vi "Experiment 19.vi"() -> ()   [LabVIEW 2026]
doc: "Experiment 19\nThis experiment is like Experiment 12 but contains 14 parallel loops (instead of 10 as in Exp 12)."
uses:
  <vilib>/AdvancedString/1D String Array to Delimited String (string).vi
  <vilib>/Analysis/baseanly.llb/Mean (DBL).vi
  <vilib>/Analysis/NI_AALBase.lvlib
panel:
  out "No. Of Iterations Executed - Loop 14":i32
  out "Output - Loop 14":dbl[](array[numeric]) format="%.3f"
  out "No. Of Iterations Executed - Loop 13":i32
  out "Output - Loop 13":dbl[](array[numeric]) format="%.3f"
  out "No. Of Iterations Executed - Loop 12":i32
  out "Output - Loop 12":dbl[](array[numeric]) format="%.3f"
  out "No. Of Iterations Executed - Loop 11":i32
  out "Output - Loop 11":dbl[](array[numeric]) format="%.3f"
  out "No. Of Iterations As Block Of Text (easy to copy into Excel)":string
  out "No. Of Iterations Executed - Loop 10":i32
  out "Output - Loop 10":dbl[](array[numeric]) format="%.3f"
  out "No. Of Iterations Executed - Loop 9":i32
  out "Output - Loop 9":dbl[](array[numeric]) format="%.3f"
  out "No. Of Iterations Executed - Loop 8":i32
  out "Output - Loop 8":dbl[](array[numeric]) format="%.3f"
  out "No. Of Iterations Executed - Loop 7":i32
  out "Output - Loop 7":dbl[](array[numeric]) format="%.3f"
  out "No. Of Iterations Executed - Loop 6":i32
  out "Output - Loop 6":dbl[](array[numeric]) format="%.3f"
  out "No. Of Iterations Executed - Loop 5":i32
  out "Output - Loop 5":dbl[](array[numeric]) format="%.3f"
  out "No. Of Iterations Executed - Loop 4":i32
  out "Output - Loop 4":dbl[](array[numeric]) format="%.3f"
  out "No. Of Iterations Executed - Loop 3":i32
  out "Output - Loop 3":dbl[](array[numeric]) format="%.3f"
  out "Avg. No. Of Iterations Executed - All Loops":dbl format="%.1f"
  out "No. Of Iterations Executed - Loop 2":i32
  out "Output - Loop 2":dbl[](array[numeric]) format="%.3f"
  out "No. Of Iterations Executed - Loop 1":i32
  out "Output - Loop 1":dbl[](array[numeric]) format="%.3f"
  out "Stop VI?":bool
  # "Experiment 19"
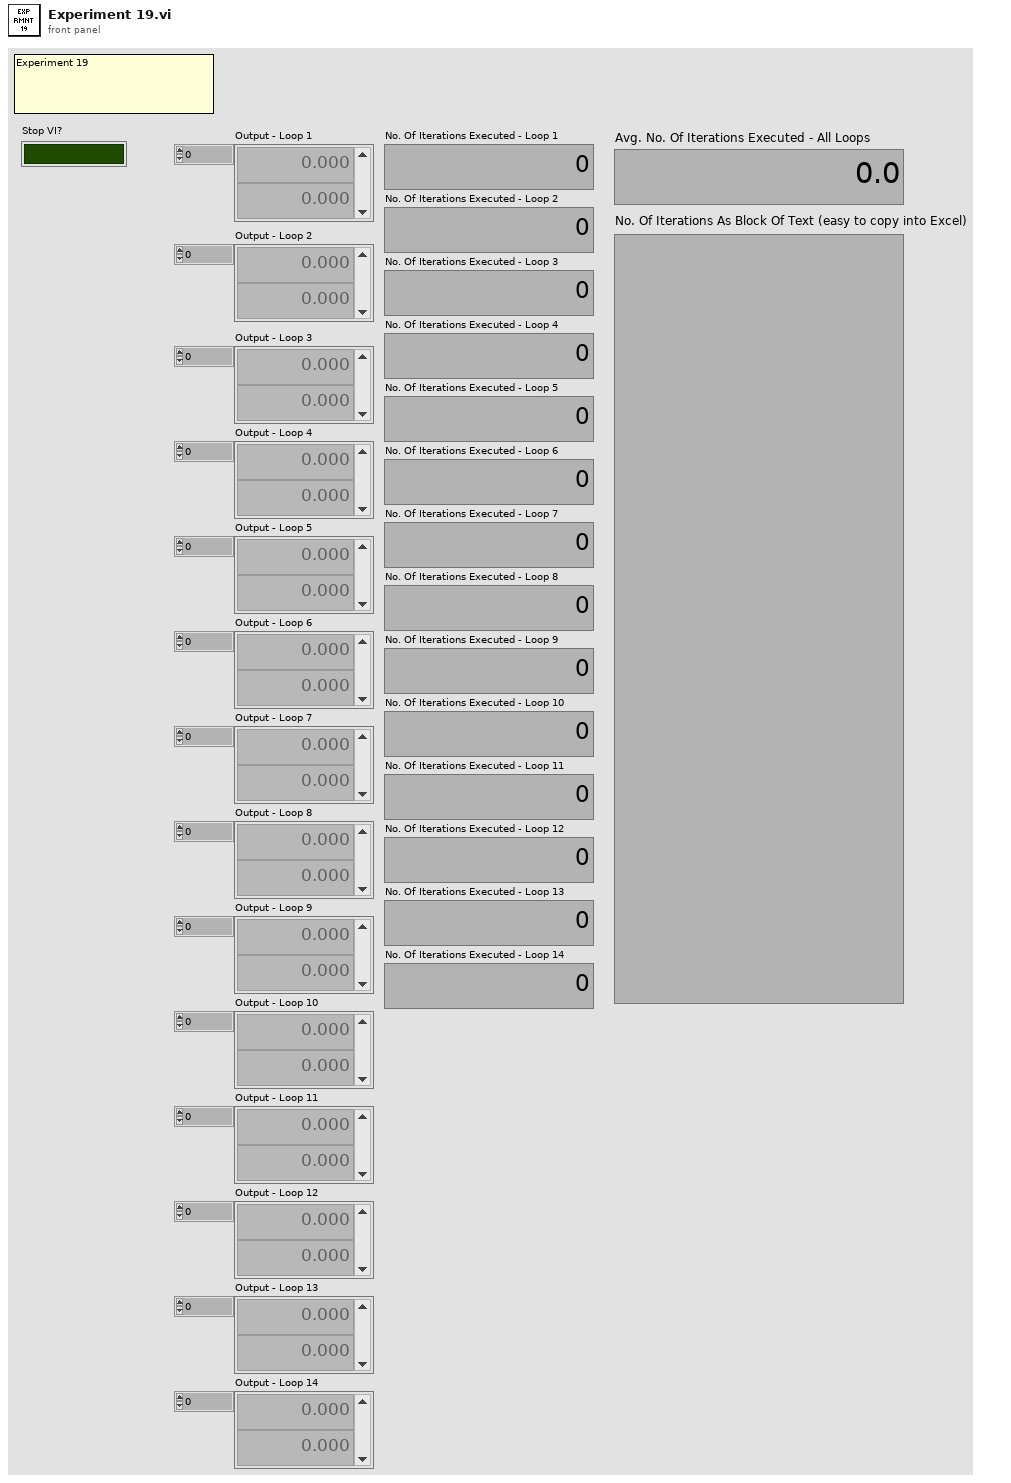
[diagram p1: front panel]
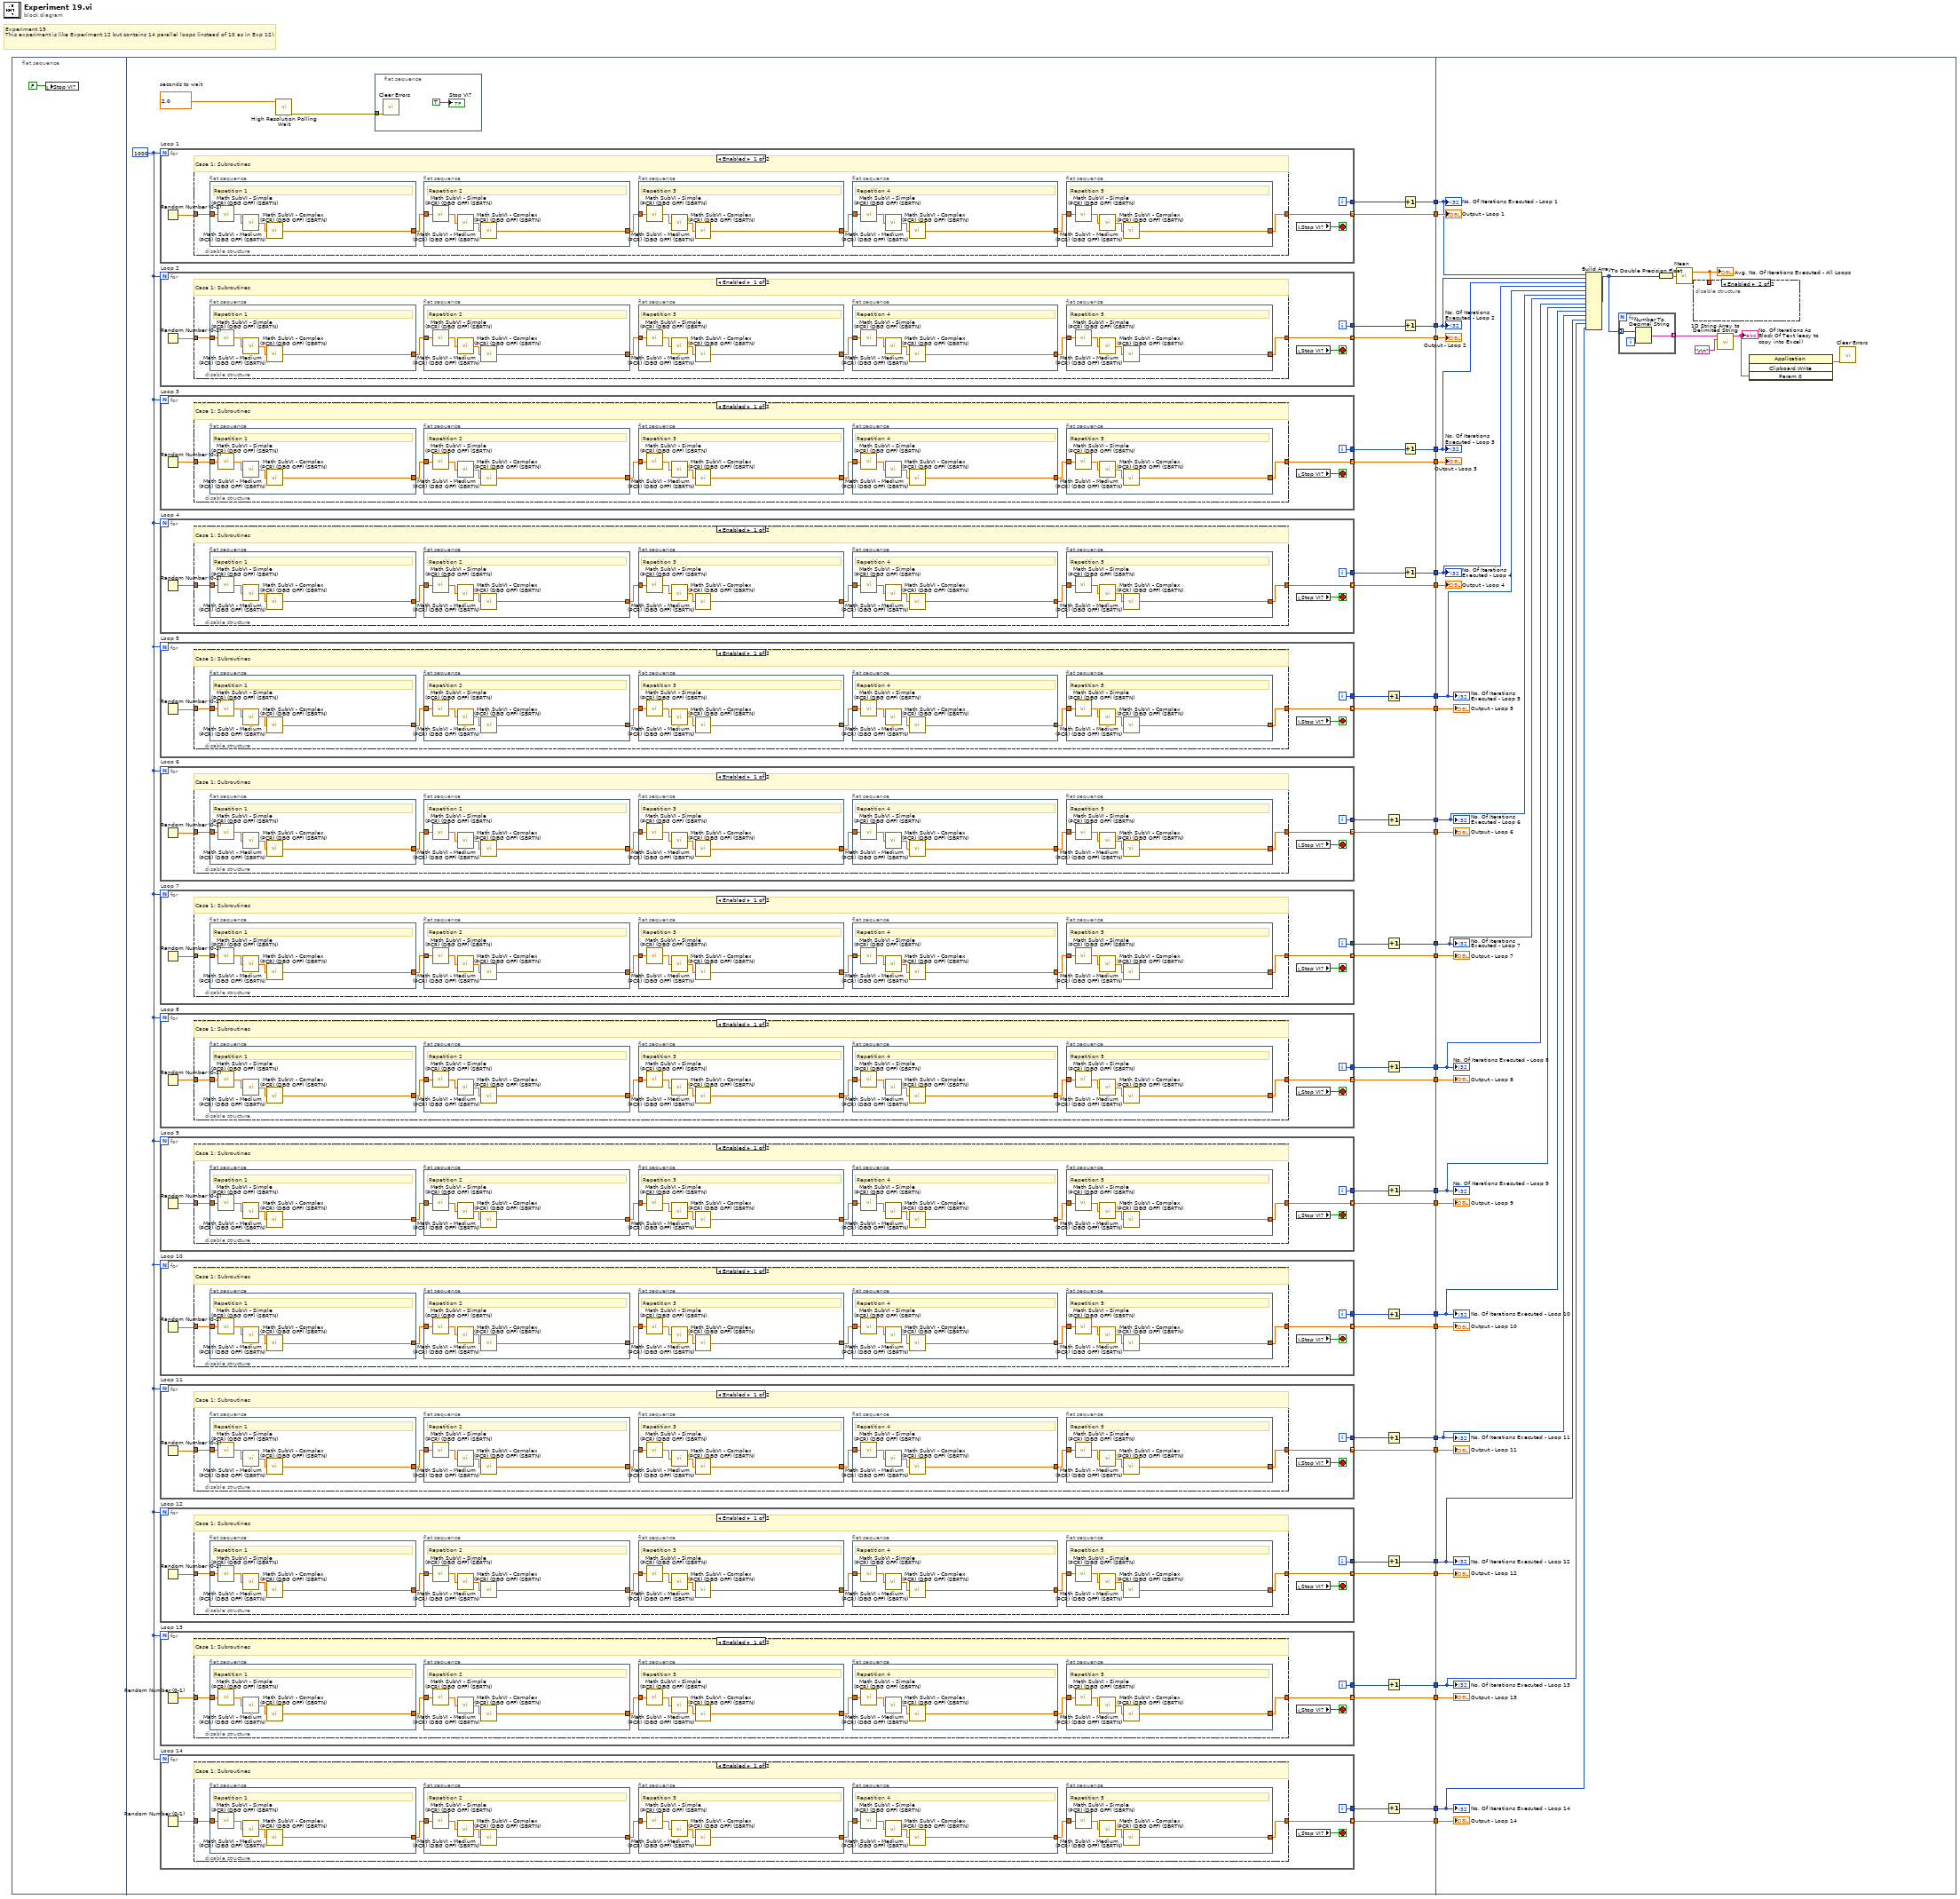
[diagram p0: block diagram]
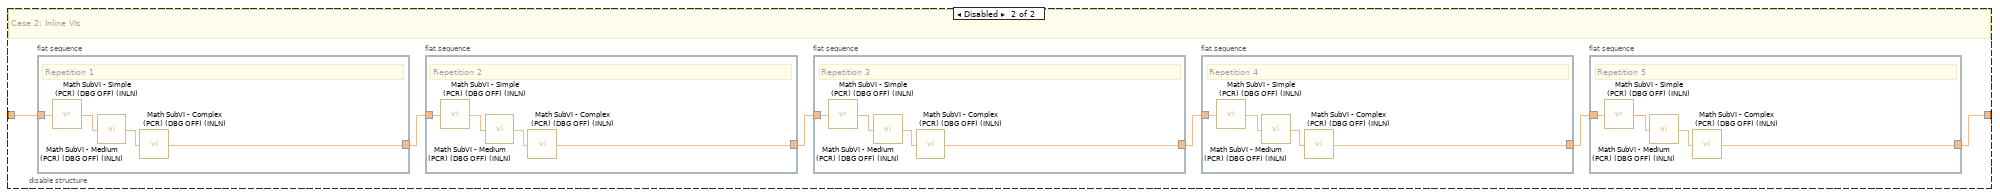
[diagram p2: hidden frame]
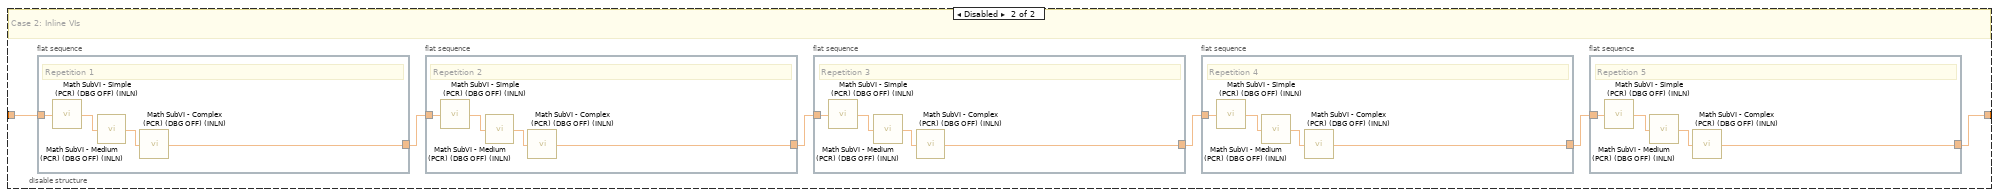
[diagram p3: hidden frame]
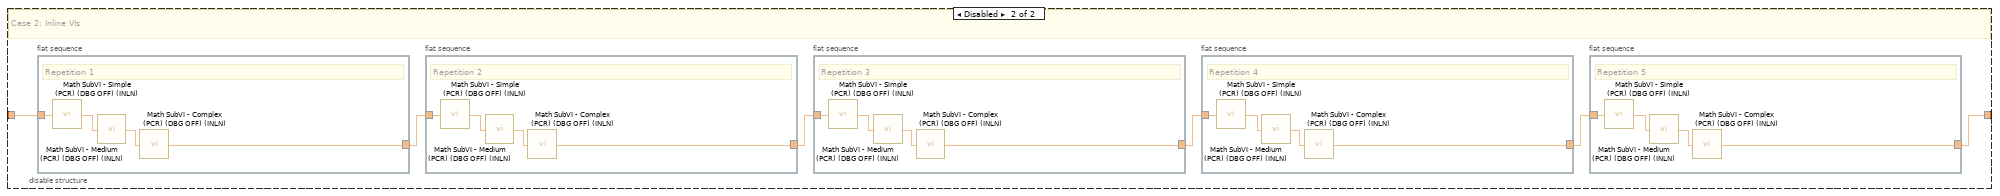
[diagram p4: hidden frame]
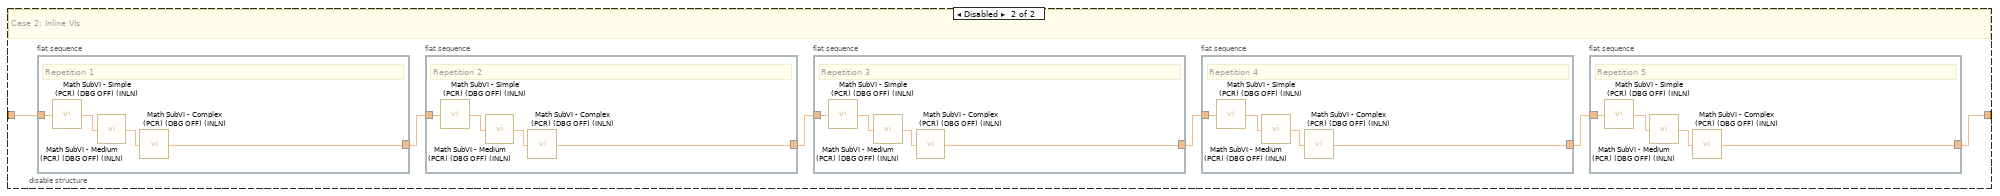
[diagram p5: hidden frame]
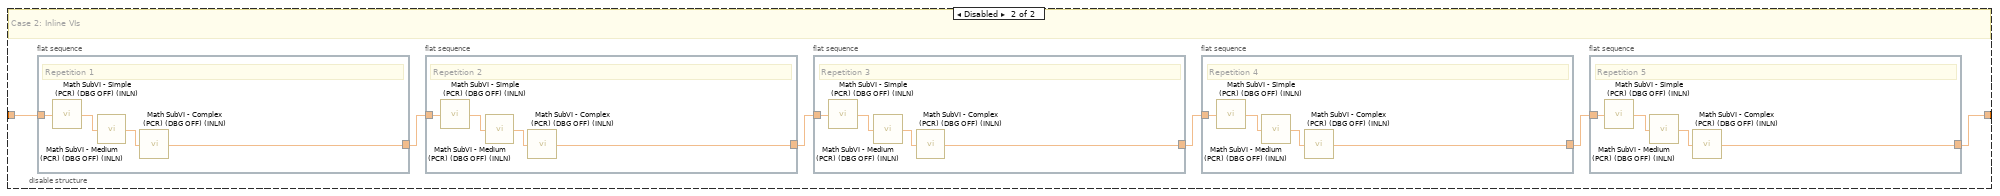
[diagram p6: hidden frame]
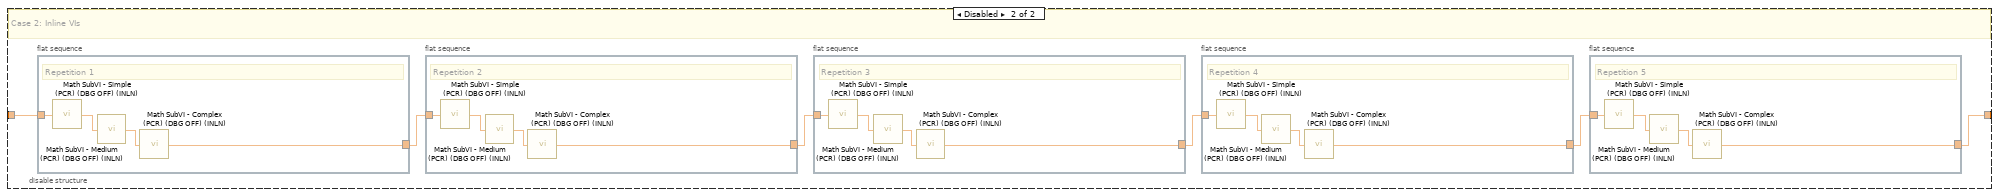
[diagram p7: hidden frame]
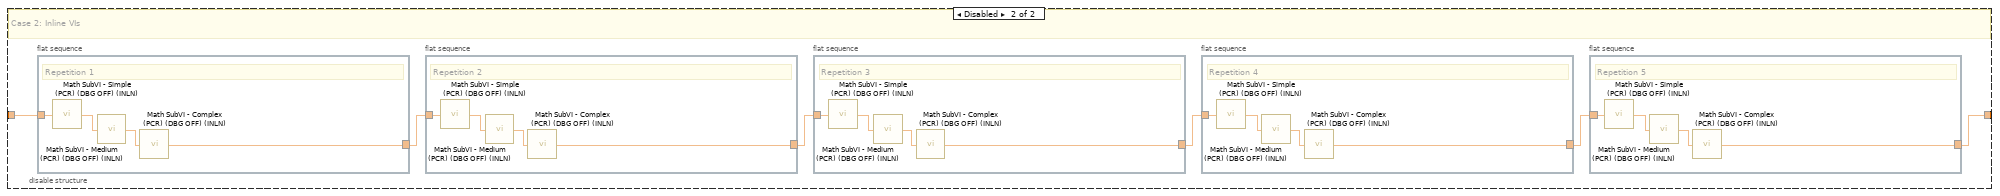
[diagram p8: hidden frame]
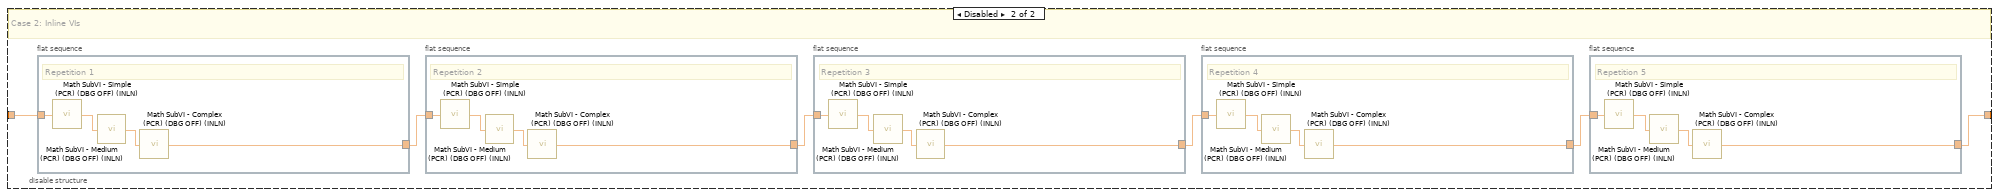
[diagram p9: hidden frame]
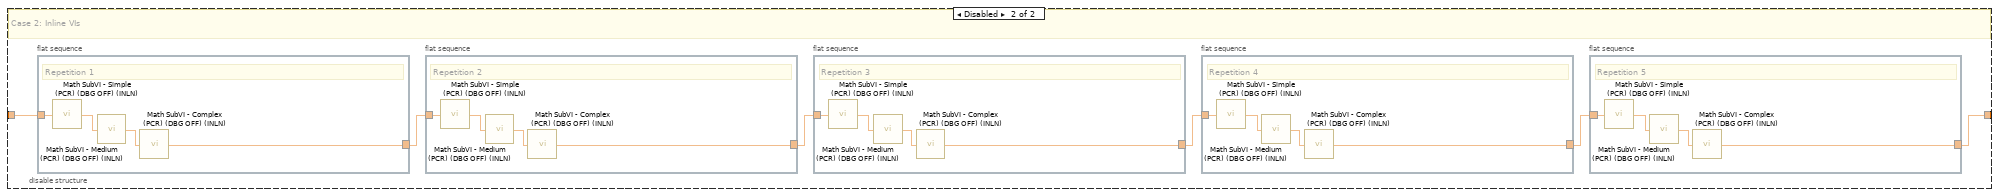
[diagram p10: hidden frame]
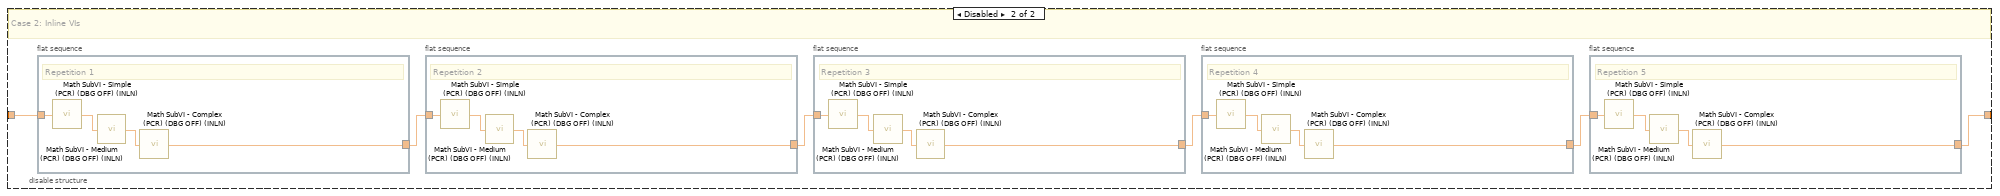
[diagram p11: hidden frame]
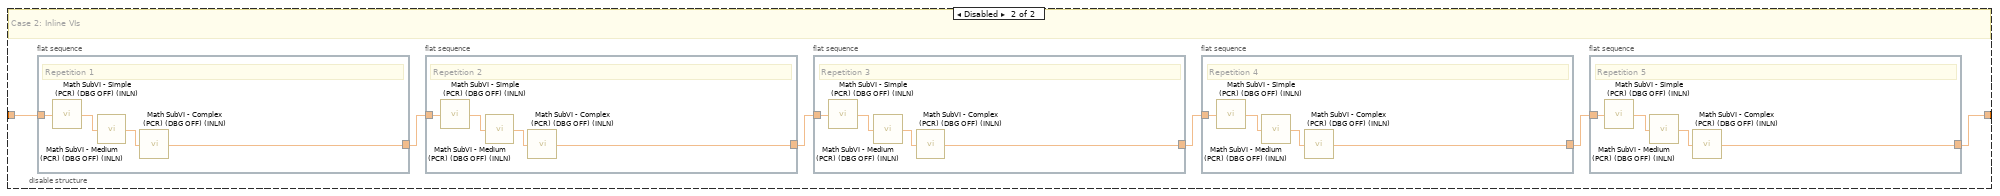
[diagram p12: hidden frame]
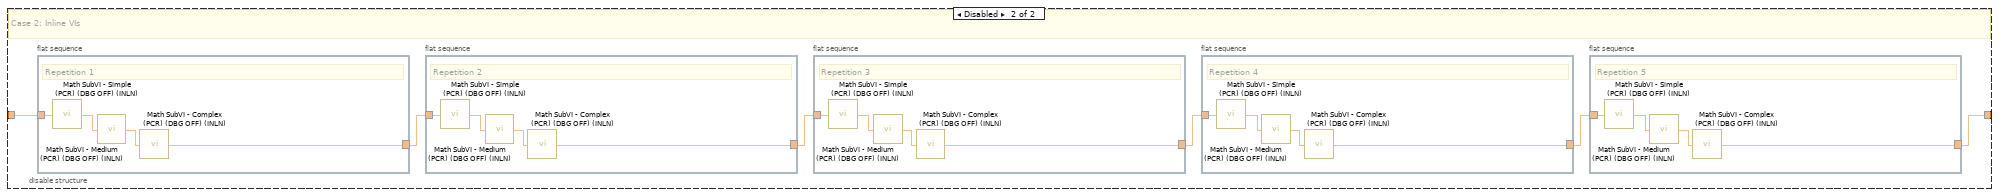
[diagram p13: hidden frame]
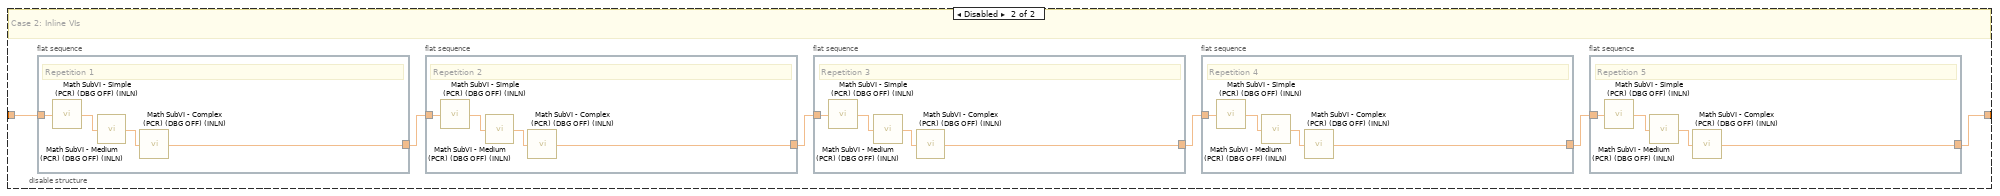
[diagram p14: hidden frame]
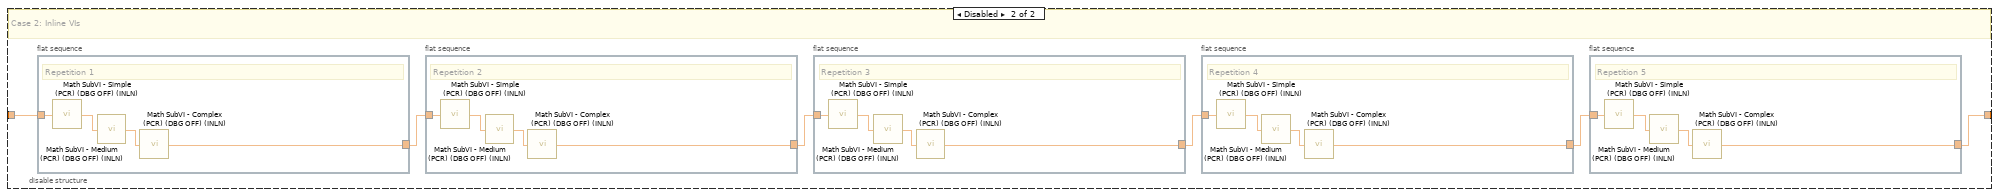
[diagram p15: hidden frame]
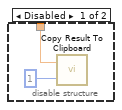
[diagram p16: hidden frame]
diagram:
  # "Experiment 19\nThis experiment is like Experiment 12 but contains 14 parallel loops (instead of 10 as in Exp 12)."
  n1 = flat-sequence {
    tunnel: [w72] -> w28
    tunnel: [w70] -> w27
    tunnel: [w69] -> w26
    tunnel: [w60] -> w25
    tunnel: [w68] -> w24
    tunnel: [w58] -> w23
    tunnel: [w56] -> w22
    tunnel: [w67] -> w21
    tunnel: [w54] -> w20
    tunnel: [w66] -> w19
    tunnel: [w52] -> w18
    tunnel: [w61] -> w17
    tunnel: [w50] -> w16
    tunnel: [w62] -> w15
    tunnel: [w47] -> w14
    tunnel: [w63] -> w13
    tunnel: [w45] -> w12
    tunnel: [w64] -> w11
    tunnel: [w43] -> w10
    tunnel: [w65] -> w9
    tunnel: [w41] -> w8
    tunnel: [w39] -> w7
    tunnel: [w38] -> w6
    tunnel: [w32] -> w5
    tunnel: [w36] -> w4
    tunnel: [w31] -> w3
    tunnel: [w34] -> w2
    tunnel: [w30] -> w1
    tunnel: w28 -> [w895]
    tunnel: w27 -> [w893]
    tunnel: w26 -> [w892]
    tunnel: w25 -> [w894]
    tunnel: w24 -> [w888]
    tunnel: w23 -> [w890]
    tunnel: w22 -> [w889]
    tunnel: w21 -> [w887]
    tunnel: w20 -> [w885]
    tunnel: w19 -> [w879]
    tunnel: w18 -> [w884]
    tunnel: w17 -> [w878]
    tunnel: w16 -> [w883]
    tunnel: w15 -> [w877]
    tunnel: w14 -> [w882]
    tunnel: w13 -> [w876]
    tunnel: w12 -> [w881]
    tunnel: w11 -> [w875]
    tunnel: w10 -> [w880]
    tunnel: w9 -> [w874]
    tunnel: w8 -> [w868]
    tunnel: w7 -> [w864]
    tunnel: w6 -> [w867]
    tunnel: w5 -> [w863]
    tunnel: w4 -> [w866]
    tunnel: w3 -> [w862]
    tunnel: w2 -> [w865]
    tunnel: w1 -> [w861]
    frame #0 {
      n2 = local write "Stop VI?"(FALSE) -> ()
    }
    frame #1 {
      w42 = 10000000
      w74 = 2.0  # seconds to wait
      n3 = for "Loop 1" {
        N: w42 -> [_]
        tunnel: [w806] -> w72 mode=indexing
        tunnel: [w807] -> w71
        i -> [w807]
        stop <- w808 stop-if-true
        n4 = Random Number (0-1)() -> (number: 0 to 1=w805:dbl)
        n5 = disable-structure shown="Enabled" {
          disable-tunnel: w805 -> [w814 w840]
          disable-tunnel: [w813 w835] -> w806
          frame Enabled {
            # "Case 1: Subroutines"
            n6 = flat-sequence {
              tunnel: w814 -> [w834]
              tunnel: [w831] -> w809
              frame #0 {
                # "Repetition 1"
                n7 = call "Math SubVI - Simple (PCR) (DBG OFF) (SBRTN).vi"("Input"=w834) -> ("Output"=w832:dbl)
                n8 = call "Math SubVI - Medium (PCR) (DBG OFF) (SBRTN).vi"("Input"=w832) -> ("Output"=w833:dbl)
                n9 = call "Math SubVI - Complex (PCR) (DBG OFF) (SBRTN).vi"("Input"=w833) -> ("Output"=w831:dbl)
              }
            }
            n10 = flat-sequence {
              tunnel: w809 -> [w830]
              tunnel: [w827] -> w812
              frame #0 {
                # "Repetition 2"
                n11 = call "Math SubVI - Simple (PCR) (DBG OFF) (SBRTN).vi"("Input"=w830) -> ("Output"=w828:dbl)
                n12 = call "Math SubVI - Medium (PCR) (DBG OFF) (SBRTN).vi"("Input"=w828) -> ("Output"=w829:dbl)
                n13 = call "Math SubVI - Complex (PCR) (DBG OFF) (SBRTN).vi"("Input"=w829) -> ("Output"=w827:dbl)
              }
            }
            n14 = flat-sequence {
              tunnel: w812 -> [w826]
              tunnel: [w823] -> w811
              frame #0 {
                # "Repetition 3"
                n15 = call "Math SubVI - Simple (PCR) (DBG OFF) (SBRTN).vi"("Input"=w826) -> ("Output"=w824:dbl)
                n16 = call "Math SubVI - Medium (PCR) (DBG OFF) (SBRTN).vi"("Input"=w824) -> ("Output"=w825:dbl)
                n17 = call "Math SubVI - Complex (PCR) (DBG OFF) (SBRTN).vi"("Input"=w825) -> ("Output"=w823:dbl)
              }
            }
            n18 = flat-sequence {
              tunnel: w811 -> [w822]
              tunnel: [w819] -> w810
              frame #0 {
                # "Repetition 4"
                n19 = call "Math SubVI - Simple (PCR) (DBG OFF) (SBRTN).vi"("Input"=w822) -> ("Output"=w820:dbl)
                n20 = call "Math SubVI - Medium (PCR) (DBG OFF) (SBRTN).vi"("Input"=w820) -> ("Output"=w821:dbl)
                n21 = call "Math SubVI - Complex (PCR) (DBG OFF) (SBRTN).vi"("Input"=w821) -> ("Output"=w819:dbl)
              }
            }
            n22 = flat-sequence {
              tunnel: w810 -> [w818]
              tunnel: [w815] -> w813
              frame #0 {
                # "Repetition 5"
                n23 = call "Math SubVI - Simple (PCR) (DBG OFF) (SBRTN).vi"("Input"=w818) -> ("Output"=w816:dbl)
                n24 = call "Math SubVI - Medium (PCR) (DBG OFF) (SBRTN).vi"("Input"=w816) -> ("Output"=w817:dbl)
                n25 = call "Math SubVI - Complex (PCR) (DBG OFF) (SBRTN).vi"("Input"=w817) -> ("Output"=w815:dbl)
              }
            }
          }
          frame Disabled {
            # "Case 2: Inline VIs"
            n26 = flat-sequence {
              tunnel: w840 -> [w860]
              tunnel: [w857] -> w839
              frame #0 {
                # "Repetition 1"
                n27 = call "Math SubVI - Simple (PCR) (DBG OFF) (INLN).vi"("Input"=w860) -> ("Output"=w858:dbl)
                n28 = call "Math SubVI - Medium (PCR) (DBG OFF) (INLN).vi"("Input"=w858) -> ("Output"=w859:dbl)
                n29 = call "Math SubVI - Complex (PCR) (DBG OFF) (INLN).vi"("Input"=w859) -> ("Output"=w857:dbl)
              }
            }
            n30 = flat-sequence {
              tunnel: w839 -> [w856]
              tunnel: [w853] -> w838
              frame #0 {
                # "Repetition 2"
                n31 = call "Math SubVI - Simple (PCR) (DBG OFF) (INLN).vi"("Input"=w856) -> ("Output"=w854:dbl)
                n32 = call "Math SubVI - Medium (PCR) (DBG OFF) (INLN).vi"("Input"=w854) -> ("Output"=w855:dbl)
                n33 = call "Math SubVI - Complex (PCR) (DBG OFF) (INLN).vi"("Input"=w855) -> ("Output"=w853:dbl)
              }
            }
            n34 = flat-sequence {
              tunnel: w838 -> [w852]
              tunnel: [w849] -> w837
              frame #0 {
                # "Repetition 3"
                n35 = call "Math SubVI - Simple (PCR) (DBG OFF) (INLN).vi"("Input"=w852) -> ("Output"=w850:dbl)
                n36 = call "Math SubVI - Medium (PCR) (DBG OFF) (INLN).vi"("Input"=w850) -> ("Output"=w851:dbl)
                n37 = call "Math SubVI - Complex (PCR) (DBG OFF) (INLN).vi"("Input"=w851) -> ("Output"=w849:dbl)
              }
            }
            n38 = flat-sequence {
              tunnel: w837 -> [w848]
              tunnel: [w845] -> w836
              frame #0 {
                # "Repetition 4"
                n39 = call "Math SubVI - Simple (PCR) (DBG OFF) (INLN).vi"("Input"=w848) -> ("Output"=w846:dbl)
                n40 = call "Math SubVI - Medium (PCR) (DBG OFF) (INLN).vi"("Input"=w846) -> ("Output"=w847:dbl)
                n41 = call "Math SubVI - Complex (PCR) (DBG OFF) (INLN).vi"("Input"=w847) -> ("Output"=w845:dbl)
              }
            }
            n42 = flat-sequence {
              tunnel: w836 -> [w844]
              tunnel: [w841] -> w835
              frame #0 {
                # "Repetition 5"
                n43 = call "Math SubVI - Simple (PCR) (DBG OFF) (INLN).vi"("Input"=w844) -> ("Output"=w842:dbl)
                n44 = call "Math SubVI - Medium (PCR) (DBG OFF) (INLN).vi"("Input"=w842) -> ("Output"=w843:dbl)
                n45 = call "Math SubVI - Complex (PCR) (DBG OFF) (INLN).vi"("Input"=w843) -> ("Output"=w841:dbl)
              }
            }
          }
        }
        n46 = local read "Stop VI?"() -> (w808:bool)
      }
      n47 = for "Loop 2" {
        N: w42 -> [_]
        tunnel: [w750] -> w60 mode=indexing
        tunnel: [w751] -> w59
        i -> [w751]
        stop <- w752 stop-if-true
        n48 = Random Number (0-1)() -> (number: 0 to 1=w749:dbl)
        n49 = disable-structure shown="Enabled" {
          disable-tunnel: w749 -> [w758 w784]
          disable-tunnel: [w757 w779] -> w750
          frame Enabled {
            # "Case 1: Subroutines"
            n50 = flat-sequence {
              tunnel: w758 -> [w778]
              tunnel: [w775] -> w753
              frame #0 {
                # "Repetition 1"
                n51 = call "Math SubVI - Simple (PCR) (DBG OFF) (SBRTN).vi"("Input"=w778) -> ("Output"=w776:dbl)
                n52 = call "Math SubVI - Medium (PCR) (DBG OFF) (SBRTN).vi"("Input"=w776) -> ("Output"=w777:dbl)
                n53 = call "Math SubVI - Complex (PCR) (DBG OFF) (SBRTN).vi"("Input"=w777) -> ("Output"=w775:dbl)
              }
            }
            n54 = flat-sequence {
              tunnel: w753 -> [w774]
              tunnel: [w771] -> w756
              frame #0 {
                # "Repetition 2"
                n55 = call "Math SubVI - Simple (PCR) (DBG OFF) (SBRTN).vi"("Input"=w774) -> ("Output"=w772:dbl)
                n56 = call "Math SubVI - Medium (PCR) (DBG OFF) (SBRTN).vi"("Input"=w772) -> ("Output"=w773:dbl)
                n57 = call "Math SubVI - Complex (PCR) (DBG OFF) (SBRTN).vi"("Input"=w773) -> ("Output"=w771:dbl)
              }
            }
            n58 = flat-sequence {
              tunnel: w756 -> [w770]
              tunnel: [w767] -> w755
              frame #0 {
                # "Repetition 3"
                n59 = call "Math SubVI - Simple (PCR) (DBG OFF) (SBRTN).vi"("Input"=w770) -> ("Output"=w768:dbl)
                n60 = call "Math SubVI - Medium (PCR) (DBG OFF) (SBRTN).vi"("Input"=w768) -> ("Output"=w769:dbl)
                n61 = call "Math SubVI - Complex (PCR) (DBG OFF) (SBRTN).vi"("Input"=w769) -> ("Output"=w767:dbl)
              }
            }
            n62 = flat-sequence {
              tunnel: w755 -> [w766]
              tunnel: [w763] -> w754
              frame #0 {
                # "Repetition 4"
                n63 = call "Math SubVI - Simple (PCR) (DBG OFF) (SBRTN).vi"("Input"=w766) -> ("Output"=w764:dbl)
                n64 = call "Math SubVI - Medium (PCR) (DBG OFF) (SBRTN).vi"("Input"=w764) -> ("Output"=w765:dbl)
                n65 = call "Math SubVI - Complex (PCR) (DBG OFF) (SBRTN).vi"("Input"=w765) -> ("Output"=w763:dbl)
              }
            }
            n66 = flat-sequence {
              tunnel: w754 -> [w762]
              tunnel: [w759] -> w757
              frame #0 {
                # "Repetition 5"
                n67 = call "Math SubVI - Simple (PCR) (DBG OFF) (SBRTN).vi"("Input"=w762) -> ("Output"=w760:dbl)
                n68 = call "Math SubVI - Medium (PCR) (DBG OFF) (SBRTN).vi"("Input"=w760) -> ("Output"=w761:dbl)
                n69 = call "Math SubVI - Complex (PCR) (DBG OFF) (SBRTN).vi"("Input"=w761) -> ("Output"=w759:dbl)
              }
            }
          }
          frame Disabled {
            # "Case 2: Inline VIs"
            n70 = flat-sequence {
              tunnel: w784 -> [w804]
              tunnel: [w801] -> w783
              frame #0 {
                # "Repetition 1"
                n71 = call "Math SubVI - Simple (PCR) (DBG OFF) (INLN).vi"("Input"=w804) -> ("Output"=w802:dbl)
                n72 = call "Math SubVI - Medium (PCR) (DBG OFF) (INLN).vi"("Input"=w802) -> ("Output"=w803:dbl)
                n73 = call "Math SubVI - Complex (PCR) (DBG OFF) (INLN).vi"("Input"=w803) -> ("Output"=w801:dbl)
              }
            }
            n74 = flat-sequence {
              tunnel: w783 -> [w800]
              tunnel: [w797] -> w782
              frame #0 {
                # "Repetition 2"
                n75 = call "Math SubVI - Simple (PCR) (DBG OFF) (INLN).vi"("Input"=w800) -> ("Output"=w798:dbl)
                n76 = call "Math SubVI - Medium (PCR) (DBG OFF) (INLN).vi"("Input"=w798) -> ("Output"=w799:dbl)
                n77 = call "Math SubVI - Complex (PCR) (DBG OFF) (INLN).vi"("Input"=w799) -> ("Output"=w797:dbl)
              }
            }
            n78 = flat-sequence {
              tunnel: w782 -> [w796]
              tunnel: [w793] -> w781
              frame #0 {
                # "Repetition 3"
                n79 = call "Math SubVI - Simple (PCR) (DBG OFF) (INLN).vi"("Input"=w796) -> ("Output"=w794:dbl)
                n80 = call "Math SubVI - Medium (PCR) (DBG OFF) (INLN).vi"("Input"=w794) -> ("Output"=w795:dbl)
                n81 = call "Math SubVI - Complex (PCR) (DBG OFF) (INLN).vi"("Input"=w795) -> ("Output"=w793:dbl)
              }
            }
            n82 = flat-sequence {
              tunnel: w781 -> [w792]
              tunnel: [w789] -> w780
              frame #0 {
                # "Repetition 4"
                n83 = call "Math SubVI - Simple (PCR) (DBG OFF) (INLN).vi"("Input"=w792) -> ("Output"=w790:dbl)
                n84 = call "Math SubVI - Medium (PCR) (DBG OFF) (INLN).vi"("Input"=w790) -> ("Output"=w791:dbl)
                n85 = call "Math SubVI - Complex (PCR) (DBG OFF) (INLN).vi"("Input"=w791) -> ("Output"=w789:dbl)
              }
            }
            n86 = flat-sequence {
              tunnel: w780 -> [w788]
              tunnel: [w785] -> w779
              frame #0 {
                # "Repetition 5"
                n87 = call "Math SubVI - Simple (PCR) (DBG OFF) (INLN).vi"("Input"=w788) -> ("Output"=w786:dbl)
                n88 = call "Math SubVI - Medium (PCR) (DBG OFF) (INLN).vi"("Input"=w786) -> ("Output"=w787:dbl)
                n89 = call "Math SubVI - Complex (PCR) (DBG OFF) (INLN).vi"("Input"=w787) -> ("Output"=w785:dbl)
              }
            }
          }
        }
        n90 = local read "Stop VI?"() -> (w752:bool)
      }
      n91 = for "Loop 3" {
        N: w42 -> [_]
        tunnel: [w694] -> w58 mode=indexing
        tunnel: [w695] -> w57
        i -> [w695]
        stop <- w696 stop-if-true
        n92 = Random Number (0-1)() -> (number: 0 to 1=w693:dbl)
        n93 = disable-structure shown="Enabled" {
          disable-tunnel: w693 -> [w702 w728]
          disable-tunnel: [w701 w723] -> w694
          frame Enabled {
            # "Case 1: Subroutines"
            n94 = flat-sequence {
              tunnel: w702 -> [w722]
              tunnel: [w719] -> w697
              frame #0 {
                # "Repetition 1"
                n95 = call "Math SubVI - Simple (PCR) (DBG OFF) (SBRTN).vi"("Input"=w722) -> ("Output"=w720:dbl)
                n96 = call "Math SubVI - Medium (PCR) (DBG OFF) (SBRTN).vi"("Input"=w720) -> ("Output"=w721:dbl)
                n97 = call "Math SubVI - Complex (PCR) (DBG OFF) (SBRTN).vi"("Input"=w721) -> ("Output"=w719:dbl)
              }
            }
            n98 = flat-sequence {
              tunnel: w697 -> [w718]
              tunnel: [w715] -> w700
              frame #0 {
                # "Repetition 2"
                n99 = call "Math SubVI - Simple (PCR) (DBG OFF) (SBRTN).vi"("Input"=w718) -> ("Output"=w716:dbl)
                n100 = call "Math SubVI - Medium (PCR) (DBG OFF) (SBRTN).vi"("Input"=w716) -> ("Output"=w717:dbl)
                n101 = call "Math SubVI - Complex (PCR) (DBG OFF) (SBRTN).vi"("Input"=w717) -> ("Output"=w715:dbl)
              }
            }
            n102 = flat-sequence {
              tunnel: w700 -> [w714]
              tunnel: [w711] -> w699
              frame #0 {
                # "Repetition 3"
                n103 = call "Math SubVI - Simple (PCR) (DBG OFF) (SBRTN).vi"("Input"=w714) -> ("Output"=w712:dbl)
                n104 = call "Math SubVI - Medium (PCR) (DBG OFF) (SBRTN).vi"("Input"=w712) -> ("Output"=w713:dbl)
                n105 = call "Math SubVI - Complex (PCR) (DBG OFF) (SBRTN).vi"("Input"=w713) -> ("Output"=w711:dbl)
              }
            }
            n106 = flat-sequence {
              tunnel: w699 -> [w710]
              tunnel: [w707] -> w698
              frame #0 {
                # "Repetition 4"
                n107 = call "Math SubVI - Simple (PCR) (DBG OFF) (SBRTN).vi"("Input"=w710) -> ("Output"=w708:dbl)
                n108 = call "Math SubVI - Medium (PCR) (DBG OFF) (SBRTN).vi"("Input"=w708) -> ("Output"=w709:dbl)
                n109 = call "Math SubVI - Complex (PCR) (DBG OFF) (SBRTN).vi"("Input"=w709) -> ("Output"=w707:dbl)
              }
            }
            n110 = flat-sequence {
              tunnel: w698 -> [w706]
              tunnel: [w703] -> w701
              frame #0 {
                # "Repetition 5"
                n111 = call "Math SubVI - Simple (PCR) (DBG OFF) (SBRTN).vi"("Input"=w706) -> ("Output"=w704:dbl)
                n112 = call "Math SubVI - Medium (PCR) (DBG OFF) (SBRTN).vi"("Input"=w704) -> ("Output"=w705:dbl)
                n113 = call "Math SubVI - Complex (PCR) (DBG OFF) (SBRTN).vi"("Input"=w705) -> ("Output"=w703:dbl)
              }
            }
          }
          frame Disabled {
            # "Case 2: Inline VIs"
            n114 = flat-sequence {
              tunnel: w728 -> [w748]
              tunnel: [w745] -> w727
              frame #0 {
                # "Repetition 1"
                n115 = call "Math SubVI - Simple (PCR) (DBG OFF) (INLN).vi"("Input"=w748) -> ("Output"=w746:dbl)
                n116 = call "Math SubVI - Medium (PCR) (DBG OFF) (INLN).vi"("Input"=w746) -> ("Output"=w747:dbl)
                n117 = call "Math SubVI - Complex (PCR) (DBG OFF) (INLN).vi"("Input"=w747) -> ("Output"=w745:dbl)
              }
            }
            n118 = flat-sequence {
              tunnel: w727 -> [w744]
              tunnel: [w741] -> w726
              frame #0 {
                # "Repetition 2"
                n119 = call "Math SubVI - Simple (PCR) (DBG OFF) (INLN).vi"("Input"=w744) -> ("Output"=w742:dbl)
                n120 = call "Math SubVI - Medium (PCR) (DBG OFF) (INLN).vi"("Input"=w742) -> ("Output"=w743:dbl)
                n121 = call "Math SubVI - Complex (PCR) (DBG OFF) (INLN).vi"("Input"=w743) -> ("Output"=w741:dbl)
              }
            }
            n122 = flat-sequence {
              tunnel: w726 -> [w740]
              tunnel: [w737] -> w725
              frame #0 {
                # "Repetition 3"
                n123 = call "Math SubVI - Simple (PCR) (DBG OFF) (INLN).vi"("Input"=w740) -> ("Output"=w738:dbl)
                n124 = call "Math SubVI - Medium (PCR) (DBG OFF) (INLN).vi"("Input"=w738) -> ("Output"=w739:dbl)
                n125 = call "Math SubVI - Complex (PCR) (DBG OFF) (INLN).vi"("Input"=w739) -> ("Output"=w737:dbl)
              }
            }
            n126 = flat-sequence {
              tunnel: w725 -> [w736]
              tunnel: [w733] -> w724
              frame #0 {
                # "Repetition 4"
                n127 = call "Math SubVI - Simple (PCR) (DBG OFF) (INLN).vi"("Input"=w736) -> ("Output"=w734:dbl)
                n128 = call "Math SubVI - Medium (PCR) (DBG OFF) (INLN).vi"("Input"=w734) -> ("Output"=w735:dbl)
                n129 = call "Math SubVI - Complex (PCR) (DBG OFF) (INLN).vi"("Input"=w735) -> ("Output"=w733:dbl)
              }
            }
            n130 = flat-sequence {
              tunnel: w724 -> [w732]
              tunnel: [w729] -> w723
              frame #0 {
                # "Repetition 5"
                n131 = call "Math SubVI - Simple (PCR) (DBG OFF) (INLN).vi"("Input"=w732) -> ("Output"=w730:dbl)
                n132 = call "Math SubVI - Medium (PCR) (DBG OFF) (INLN).vi"("Input"=w730) -> ("Output"=w731:dbl)
                n133 = call "Math SubVI - Complex (PCR) (DBG OFF) (INLN).vi"("Input"=w731) -> ("Output"=w729:dbl)
              }
            }
          }
        }
        n134 = local read "Stop VI?"() -> (w696:bool)
      }
      n135 = for "Loop 4" {
        N: w42 -> [_]
        tunnel: [w638] -> w56 mode=indexing
        tunnel: [w639] -> w55
        i -> [w639]
        stop <- w640 stop-if-true
        n136 = Random Number (0-1)() -> (number: 0 to 1=w637:dbl)
        n137 = disable-structure shown="Enabled" {
          disable-tunnel: w637 -> [w646 w672]
          disable-tunnel: [w645 w667] -> w638
          frame Enabled {
            # "Case 1: Subroutines"
            n138 = flat-sequence {
              tunnel: w646 -> [w666]
              tunnel: [w663] -> w641
              frame #0 {
                # "Repetition 1"
                n139 = call "Math SubVI - Simple (PCR) (DBG OFF) (SBRTN).vi"("Input"=w666) -> ("Output"=w664:dbl)
                n140 = call "Math SubVI - Medium (PCR) (DBG OFF) (SBRTN).vi"("Input"=w664) -> ("Output"=w665:dbl)
                n141 = call "Math SubVI - Complex (PCR) (DBG OFF) (SBRTN).vi"("Input"=w665) -> ("Output"=w663:dbl)
              }
            }
            n142 = flat-sequence {
              tunnel: w641 -> [w662]
              tunnel: [w659] -> w644
              frame #0 {
                # "Repetition 2"
                n143 = call "Math SubVI - Simple (PCR) (DBG OFF) (SBRTN).vi"("Input"=w662) -> ("Output"=w660:dbl)
                n144 = call "Math SubVI - Medium (PCR) (DBG OFF) (SBRTN).vi"("Input"=w660) -> ("Output"=w661:dbl)
                n145 = call "Math SubVI - Complex (PCR) (DBG OFF) (SBRTN).vi"("Input"=w661) -> ("Output"=w659:dbl)
              }
            }
            n146 = flat-sequence {
              tunnel: w644 -> [w658]
              tunnel: [w655] -> w643
              frame #0 {
                # "Repetition 3"
                n147 = call "Math SubVI - Simple (PCR) (DBG OFF) (SBRTN).vi"("Input"=w658) -> ("Output"=w656:dbl)
                n148 = call "Math SubVI - Medium (PCR) (DBG OFF) (SBRTN).vi"("Input"=w656) -> ("Output"=w657:dbl)
                n149 = call "Math SubVI - Complex (PCR) (DBG OFF) (SBRTN).vi"("Input"=w657) -> ("Output"=w655:dbl)
              }
            }
            n150 = flat-sequence {
              tunnel: w643 -> [w654]
              tunnel: [w651] -> w642
              frame #0 {
                # "Repetition 4"
                n151 = call "Math SubVI - Simple (PCR) (DBG OFF) (SBRTN).vi"("Input"=w654) -> ("Output"=w652:dbl)
                n152 = call "Math SubVI - Medium (PCR) (DBG OFF) (SBRTN).vi"("Input"=w652) -> ("Output"=w653:dbl)
                n153 = call "Math SubVI - Complex (PCR) (DBG OFF) (SBRTN).vi"("Input"=w653) -> ("Output"=w651:dbl)
              }
            }
            n154 = flat-sequence {
              tunnel: w642 -> [w650]
              tunnel: [w647] -> w645
              frame #0 {
                # "Repetition 5"
                n155 = call "Math SubVI - Simple (PCR) (DBG OFF) (SBRTN).vi"("Input"=w650) -> ("Output"=w648:dbl)
                n156 = call "Math SubVI - Medium (PCR) (DBG OFF) (SBRTN).vi"("Input"=w648) -> ("Output"=w649:dbl)
                n157 = call "Math SubVI - Complex (PCR) (DBG OFF) (SBRTN).vi"("Input"=w649) -> ("Output"=w647:dbl)
              }
            }
          }
          frame Disabled {
            # "Case 2: Inline VIs"
            n158 = flat-sequence {
              tunnel: w672 -> [w692]
              tunnel: [w689] -> w671
              frame #0 {
                # "Repetition 1"
                n159 = call "Math SubVI - Simple (PCR) (DBG OFF) (INLN).vi"("Input"=w692) -> ("Output"=w690:dbl)
                n160 = call "Math SubVI - Medium (PCR) (DBG OFF) (INLN).vi"("Input"=w690) -> ("Output"=w691:dbl)
                n161 = call "Math SubVI - Complex (PCR) (DBG OFF) (INLN).vi"("Input"=w691) -> ("Output"=w689:dbl)
              }
            }
            n162 = flat-sequence {
              tunnel: w671 -> [w688]
              tunnel: [w685] -> w670
              frame #0 {
                # "Repetition 2"
                n163 = call "Math SubVI - Simple (PCR) (DBG OFF) (INLN).vi"("Input"=w688) -> ("Output"=w686:dbl)
                n164 = call "Math SubVI - Medium (PCR) (DBG OFF) (INLN).vi"("Input"=w686) -> ("Output"=w687:dbl)
                n165 = call "Math SubVI - Complex (PCR) (DBG OFF) (INLN).vi"("Input"=w687) -> ("Output"=w685:dbl)
              }
            }
            n166 = flat-sequence {
              tunnel: w670 -> [w684]
              tunnel: [w681] -> w669
              frame #0 {
                # "Repetition 3"
                n167 = call "Math SubVI - Simple (PCR) (DBG OFF) (INLN).vi"("Input"=w684) -> ("Output"=w682:dbl)
                n168 = call "Math SubVI - Medium (PCR) (DBG OFF) (INLN).vi"("Input"=w682) -> ("Output"=w683:dbl)
                n169 = call "Math SubVI - Complex (PCR) (DBG OFF) (INLN).vi"("Input"=w683) -> ("Output"=w681:dbl)
              }
            }
            n170 = flat-sequence {
              tunnel: w669 -> [w680]
              tunnel: [w677] -> w668
              frame #0 {
                # "Repetition 4"
                n171 = call "Math SubVI - Simple (PCR) (DBG OFF) (INLN).vi"("Input"=w680) -> ("Output"=w678:dbl)
                n172 = call "Math SubVI - Medium (PCR) (DBG OFF) (INLN).vi"("Input"=w678) -> ("Output"=w679:dbl)
                n173 = call "Math SubVI - Complex (PCR) (DBG OFF) (INLN).vi"("Input"=w679) -> ("Output"=w677:dbl)
              }
            }
            n174 = flat-sequence {
              tunnel: w668 -> [w676]
              tunnel: [w673] -> w667
              frame #0 {
                # "Repetition 5"
                n175 = call "Math SubVI - Simple (PCR) (DBG OFF) (INLN).vi"("Input"=w676) -> ("Output"=w674:dbl)
                n176 = call "Math SubVI - Medium (PCR) (DBG OFF) (INLN).vi"("Input"=w674) -> ("Output"=w675:dbl)
                n177 = call "Math SubVI - Complex (PCR) (DBG OFF) (INLN).vi"("Input"=w675) -> ("Output"=w673:dbl)
              }
            }
          }
        }
        n178 = local read "Stop VI?"() -> (w640:bool)
      }
      n179 = for "Loop 5" {
        N: w42 -> [_]
        tunnel: [w582] -> w54 mode=indexing
        tunnel: [w583] -> w53
        i -> [w583]
        stop <- w584 stop-if-true
        n180 = Random Number (0-1)() -> (number: 0 to 1=w581:dbl)
        n181 = disable-structure shown="Enabled" {
          disable-tunnel: w581 -> [w590 w616]
          disable-tunnel: [w589 w611] -> w582
          frame Enabled {
            # "Case 1: Subroutines"
            n182 = flat-sequence {
              tunnel: w590 -> [w610]
              tunnel: [w607] -> w585
              frame #0 {
                # "Repetition 1"
                n183 = call "Math SubVI - Simple (PCR) (DBG OFF) (SBRTN).vi"("Input"=w610) -> ("Output"=w608:dbl)
                n184 = call "Math SubVI - Medium (PCR) (DBG OFF) (SBRTN).vi"("Input"=w608) -> ("Output"=w609:dbl)
                n185 = call "Math SubVI - Complex (PCR) (DBG OFF) (SBRTN).vi"("Input"=w609) -> ("Output"=w607:dbl)
              }
            }
            n186 = flat-sequence {
              tunnel: w585 -> [w606]
              tunnel: [w603] -> w588
              frame #0 {
                # "Repetition 2"
                n187 = call "Math SubVI - Simple (PCR) (DBG OFF) (SBRTN).vi"("Input"=w606) -> ("Output"=w604:dbl)
                n188 = call "Math SubVI - Medium (PCR) (DBG OFF) (SBRTN).vi"("Input"=w604) -> ("Output"=w605:dbl)
                n189 = call "Math SubVI - Complex (PCR) (DBG OFF) (SBRTN).vi"("Input"=w605) -> ("Output"=w603:dbl)
              }
            }
            n190 = flat-sequence {
              tunnel: w588 -> [w602]
              tunnel: [w599] -> w587
              frame #0 {
                # "Repetition 3"
                n191 = call "Math SubVI - Simple (PCR) (DBG OFF) (SBRTN).vi"("Input"=w602) -> ("Output"=w600:dbl)
                n192 = call "Math SubVI - Medium (PCR) (DBG OFF) (SBRTN).vi"("Input"=w600) -> ("Output"=w601:dbl)
                n193 = call "Math SubVI - Complex (PCR) (DBG OFF) (SBRTN).vi"("Input"=w601) -> ("Output"=w599:dbl)
              }
            }
            n194 = flat-sequence {
              tunnel: w587 -> [w598]
              tunnel: [w595] -> w586
              frame #0 {
                # "Repetition 4"
                n195 = call "Math SubVI - Simple (PCR) (DBG OFF) (SBRTN).vi"("Input"=w598) -> ("Output"=w596:dbl)
                n196 = call "Math SubVI - Medium (PCR) (DBG OFF) (SBRTN).vi"("Input"=w596) -> ("Output"=w597:dbl)
                n197 = call "Math SubVI - Complex (PCR) (DBG OFF) (SBRTN).vi"("Input"=w597) -> ("Output"=w595:dbl)
              }
            }
            n198 = flat-sequence {
              tunnel: w586 -> [w594]
              tunnel: [w591] -> w589
              frame #0 {
                # "Repetition 5"
                n199 = call "Math SubVI - Simple (PCR) (DBG OFF) (SBRTN).vi"("Input"=w594) -> ("Output"=w592:dbl)
                n200 = call "Math SubVI - Medium (PCR) (DBG OFF) (SBRTN).vi"("Input"=w592) -> ("Output"=w593:dbl)
                n201 = call "Math SubVI - Complex (PCR) (DBG OFF) (SBRTN).vi"("Input"=w593) -> ("Output"=w591:dbl)
              }
            }
          }
          frame Disabled {
            # "Case 2: Inline VIs"
            n202 = flat-sequence {
              tunnel: w616 -> [w636]
              tunnel: [w633] -> w615
              frame #0 {
                # "Repetition 1"
                n203 = call "Math SubVI - Simple (PCR) (DBG OFF) (INLN).vi"("Input"=w636) -> ("Output"=w634:dbl)
                n204 = call "Math SubVI - Medium (PCR) (DBG OFF) (INLN).vi"("Input"=w634) -> ("Output"=w635:dbl)
                n205 = call "Math SubVI - Complex (PCR) (DBG OFF) (INLN).vi"("Input"=w635) -> ("Output"=w633:dbl)
              }
            }
            n206 = flat-sequence {
              tunnel: w615 -> [w632]
              tunnel: [w629] -> w614
              frame #0 {
                # "Repetition 2"
                n207 = call "Math SubVI - Simple (PCR) (DBG OFF) (INLN).vi"("Input"=w632) -> ("Output"=w630:dbl)
                n208 = call "Math SubVI - Medium (PCR) (DBG OFF) (INLN).vi"("Input"=w630) -> ("Output"=w631:dbl)
                n209 = call "Math SubVI - Complex (PCR) (DBG OFF) (INLN).vi"("Input"=w631) -> ("Output"=w629:dbl)
              }
            }
            n210 = flat-sequence {
              tunnel: w614 -> [w628]
              tunnel: [w625] -> w613
              frame #0 {
                # "Repetition 3"
                n211 = call "Math SubVI - Simple (PCR) (DBG OFF) (INLN).vi"("Input"=w628) -> ("Output"=w626:dbl)
                n212 = call "Math SubVI - Medium (PCR) (DBG OFF) (INLN).vi"("Input"=w626) -> ("Output"=w627:dbl)
                n213 = call "Math SubVI - Complex (PCR) (DBG OFF) (INLN).vi"("Input"=w627) -> ("Output"=w625:dbl)
              }
            }
            n214 = flat-sequence {
              tunnel: w613 -> [w624]
              tunnel: [w621] -> w612
              frame #0 {
                # "Repetition 4"
                n215 = call "Math SubVI - Simple (PCR) (DBG OFF) (INLN).vi"("Input"=w624) -> ("Output"=w622:dbl)
                n216 = call "Math SubVI - Medium (PCR) (DBG OFF) (INLN).vi"("Input"=w622) -> ("Output"=w623:dbl)
                n217 = call "Math SubVI - Complex (PCR) (DBG OFF) (INLN).vi"("Input"=w623) -> ("Output"=w621:dbl)
              }
            }
            n218 = flat-sequence {
              tunnel: w612 -> [w620]
              tunnel: [w617] -> w611
              frame #0 {
                # "Repetition 5"
                n219 = call "Math SubVI - Simple (PCR) (DBG OFF) (INLN).vi"("Input"=w620) -> ("Output"=w618:dbl)
                n220 = call "Math SubVI - Medium (PCR) (DBG OFF) (INLN).vi"("Input"=w618) -> ("Output"=w619:dbl)
                n221 = call "Math SubVI - Complex (PCR) (DBG OFF) (INLN).vi"("Input"=w619) -> ("Output"=w617:dbl)
              }
            }
          }
        }
        n222 = local read "Stop VI?"() -> (w584:bool)
      }
      n223 = for "Loop 6" {
        N: w42 -> [_]
        tunnel: [w526] -> w52 mode=indexing
        tunnel: [w527] -> w51
        i -> [w527]
        stop <- w528 stop-if-true
        n224 = Random Number (0-1)() -> (number: 0 to 1=w525:dbl)
        n225 = disable-structure shown="Enabled" {
          disable-tunnel: w525 -> [w534 w560]
          disable-tunnel: [w533 w555] -> w526
          frame Enabled {
            # "Case 1: Subroutines"
            n226 = flat-sequence {
              tunnel: w534 -> [w554]
              tunnel: [w551] -> w529
              frame #0 {
                # "Repetition 1"
                n227 = call "Math SubVI - Simple (PCR) (DBG OFF) (SBRTN).vi"("Input"=w554) -> ("Output"=w552:dbl)
                n228 = call "Math SubVI - Medium (PCR) (DBG OFF) (SBRTN).vi"("Input"=w552) -> ("Output"=w553:dbl)
                n229 = call "Math SubVI - Complex (PCR) (DBG OFF) (SBRTN).vi"("Input"=w553) -> ("Output"=w551:dbl)
              }
            }
            n230 = flat-sequence {
              tunnel: w529 -> [w550]
              tunnel: [w547] -> w532
              frame #0 {
                # "Repetition 2"
                n231 = call "Math SubVI - Simple (PCR) (DBG OFF) (SBRTN).vi"("Input"=w550) -> ("Output"=w548:dbl)
                n232 = call "Math SubVI - Medium (PCR) (DBG OFF) (SBRTN).vi"("Input"=w548) -> ("Output"=w549:dbl)
                n233 = call "Math SubVI - Complex (PCR) (DBG OFF) (SBRTN).vi"("Input"=w549) -> ("Output"=w547:dbl)
              }
            }
            n234 = flat-sequence {
              tunnel: w532 -> [w546]
              tunnel: [w543] -> w531
              frame #0 {
                # "Repetition 3"
                n235 = call "Math SubVI - Simple (PCR) (DBG OFF) (SBRTN).vi"("Input"=w546) -> ("Output"=w544:dbl)
                n236 = call "Math SubVI - Medium (PCR) (DBG OFF) (SBRTN).vi"("Input"=w544) -> ("Output"=w545:dbl)
                n237 = call "Math SubVI - Complex (PCR) (DBG OFF) (SBRTN).vi"("Input"=w545) -> ("Output"=w543:dbl)
              }
            }
            n238 = flat-sequence {
              tunnel: w531 -> [w542]
              tunnel: [w539] -> w530
              frame #0 {
                # "Repetition 4"
                n239 = call "Math SubVI - Simple (PCR) (DBG OFF) (SBRTN).vi"("Input"=w542) -> ("Output"=w540:dbl)
                n240 = call "Math SubVI - Medium (PCR) (DBG OFF) (SBRTN).vi"("Input"=w540) -> ("Output"=w541:dbl)
                n241 = call "Math SubVI - Complex (PCR) (DBG OFF) (SBRTN).vi"("Input"=w541) -> ("Output"=w539:dbl)
              }
            }
            n242 = flat-sequence {
              tunnel: w530 -> [w538]
              tunnel: [w535] -> w533
              frame #0 {
                # "Repetition 5"
                n243 = call "Math SubVI - Simple (PCR) (DBG OFF) (SBRTN).vi"("Input"=w538) -> ("Output"=w536:dbl)
                n244 = call "Math SubVI - Medium (PCR) (DBG OFF) (SBRTN).vi"("Input"=w536) -> ("Output"=w537:dbl)
                n245 = call "Math SubVI - Complex (PCR) (DBG OFF) (SBRTN).vi"("Input"=w537) -> ("Output"=w535:dbl)
              }
            }
          }
          frame Disabled {
            # "Case 2: Inline VIs"
            n246 = flat-sequence {
              tunnel: w560 -> [w580]
              tunnel: [w577] -> w559
              frame #0 {
                # "Repetition 1"
                n247 = call "Math SubVI - Simple (PCR) (DBG OFF) (INLN).vi"("Input"=w580) -> ("Output"=w578:dbl)
                n248 = call "Math SubVI - Medium (PCR) (DBG OFF) (INLN).vi"("Input"=w578) -> ("Output"=w579:dbl)
                n249 = call "Math SubVI - Complex (PCR) (DBG OFF) (INLN).vi"("Input"=w579) -> ("Output"=w577:dbl)
              }
            }
            n250 = flat-sequence {
              tunnel: w559 -> [w576]
              tunnel: [w573] -> w558
              frame #0 {
                # "Repetition 2"
                n251 = call "Math SubVI - Simple (PCR) (DBG OFF) (INLN).vi"("Input"=w576) -> ("Output"=w574:dbl)
                n252 = call "Math SubVI - Medium (PCR) (DBG OFF) (INLN).vi"("Input"=w574) -> ("Output"=w575:dbl)
                n253 = call "Math SubVI - Complex (PCR) (DBG OFF) (INLN).vi"("Input"=w575) -> ("Output"=w573:dbl)
              }
            }
            n254 = flat-sequence {
              tunnel: w558 -> [w572]
              tunnel: [w569] -> w557
              frame #0 {
                # "Repetition 3"
                n255 = call "Math SubVI - Simple (PCR) (DBG OFF) (INLN).vi"("Input"=w572) -> ("Output"=w570:dbl)
                n256 = call "Math SubVI - Medium (PCR) (DBG OFF) (INLN).vi"("Input"=w570) -> ("Output"=w571:dbl)
                n257 = call "Math SubVI - Complex (PCR) (DBG OFF) (INLN).vi"("Input"=w571) -> ("Output"=w569:dbl)
              }
            }
            n258 = flat-sequence {
              tunnel: w557 -> [w568]
              tunnel: [w565] -> w556
              frame #0 {
                # "Repetition 4"
                n259 = call "Math SubVI - Simple (PCR) (DBG OFF) (INLN).vi"("Input"=w568) -> ("Output"=w566:dbl)
                n260 = call "Math SubVI - Medium (PCR) (DBG OFF) (INLN).vi"("Input"=w566) -> ("Output"=w567:dbl)
                n261 = call "Math SubVI - Complex (PCR) (DBG OFF) (INLN).vi"("Input"=w567) -> ("Output"=w565:dbl)
              }
            }
            n262 = flat-sequence {
              tunnel: w556 -> [w564]
              tunnel: [w561] -> w555
              frame #0 {
                # "Repetition 5"
                n263 = call "Math SubVI - Simple (PCR) (DBG OFF) (INLN).vi"("Input"=w564) -> ("Output"=w562:dbl)
                n264 = call "Math SubVI - Medium (PCR) (DBG OFF) (INLN).vi"("Input"=w562) -> ("Output"=w563:dbl)
                n265 = call "Math SubVI - Complex (PCR) (DBG OFF) (INLN).vi"("Input"=w563) -> ("Output"=w561:dbl)
              }
            }
          }
        }
        n266 = local read "Stop VI?"() -> (w528:bool)
      }
      n267 = for "Loop 7" {
        N: w42 -> [_]
        tunnel: [w470] -> w50 mode=indexing
        tunnel: [w471] -> w49
        i -> [w471]
        stop <- w472 stop-if-true
        n268 = Random Number (0-1)() -> (number: 0 to 1=w469:dbl)
        n269 = disable-structure shown="Enabled" {
          disable-tunnel: w469 -> [w478 w504]
          disable-tunnel: [w477 w499] -> w470
          frame Enabled {
            # "Case 1: Subroutines"
            n270 = flat-sequence {
              tunnel: w478 -> [w498]
              tunnel: [w495] -> w473
              frame #0 {
                # "Repetition 1"
                n271 = call "Math SubVI - Simple (PCR) (DBG OFF) (SBRTN).vi"("Input"=w498) -> ("Output"=w496:dbl)
                n272 = call "Math SubVI - Medium (PCR) (DBG OFF) (SBRTN).vi"("Input"=w496) -> ("Output"=w497:dbl)
                n273 = call "Math SubVI - Complex (PCR) (DBG OFF) (SBRTN).vi"("Input"=w497) -> ("Output"=w495:dbl)
              }
            }
            n274 = flat-sequence {
              tunnel: w473 -> [w494]
              tunnel: [w491] -> w476
              frame #0 {
                # "Repetition 2"
                n275 = call "Math SubVI - Simple (PCR) (DBG OFF) (SBRTN).vi"("Input"=w494) -> ("Output"=w492:dbl)
                n276 = call "Math SubVI - Medium (PCR) (DBG OFF) (SBRTN).vi"("Input"=w492) -> ("Output"=w493:dbl)
                n277 = call "Math SubVI - Complex (PCR) (DBG OFF) (SBRTN).vi"("Input"=w493) -> ("Output"=w491:dbl)
              }
            }
            n278 = flat-sequence {
              tunnel: w476 -> [w490]
              tunnel: [w487] -> w475
              frame #0 {
                # "Repetition 3"
                n279 = call "Math SubVI - Simple (PCR) (DBG OFF) (SBRTN).vi"("Input"=w490) -> ("Output"=w488:dbl)
                n280 = call "Math SubVI - Medium (PCR) (DBG OFF) (SBRTN).vi"("Input"=w488) -> ("Output"=w489:dbl)
                n281 = call "Math SubVI - Complex (PCR) (DBG OFF) (SBRTN).vi"("Input"=w489) -> ("Output"=w487:dbl)
              }
            }
            n282 = flat-sequence {
              tunnel: w475 -> [w486]
              tunnel: [w483] -> w474
              frame #0 {
                # "Repetition 4"
                n283 = call "Math SubVI - Simple (PCR) (DBG OFF) (SBRTN).vi"("Input"=w486) -> ("Output"=w484:dbl)
                n284 = call "Math SubVI - Medium (PCR) (DBG OFF) (SBRTN).vi"("Input"=w484) -> ("Output"=w485:dbl)
                n285 = call "Math SubVI - Complex (PCR) (DBG OFF) (SBRTN).vi"("Input"=w485) -> ("Output"=w483:dbl)
              }
            }
            n286 = flat-sequence {
              tunnel: w474 -> [w482]
              tunnel: [w479] -> w477
              frame #0 {
                # "Repetition 5"
                n287 = call "Math SubVI - Simple (PCR) (DBG OFF) (SBRTN).vi"("Input"=w482) -> ("Output"=w480:dbl)
                n288 = call "Math SubVI - Medium (PCR) (DBG OFF) (SBRTN).vi"("Input"=w480) -> ("Output"=w481:dbl)
                n289 = call "Math SubVI - Complex (PCR) (DBG OFF) (SBRTN).vi"("Input"=w481) -> ("Output"=w479:dbl)
              }
            }
          }
          frame Disabled {
            # "Case 2: Inline VIs"
            n290 = flat-sequence {
              tunnel: w504 -> [w524]
              tunnel: [w521] -> w503
              frame #0 {
                # "Repetition 1"
                n291 = call "Math SubVI - Simple (PCR) (DBG OFF) (INLN).vi"("Input"=w524) -> ("Output"=w522:dbl)
                n292 = call "Math SubVI - Medium (PCR) (DBG OFF) (INLN).vi"("Input"=w522) -> ("Output"=w523:dbl)
                n293 = call "Math SubVI - Complex (PCR) (DBG OFF) (INLN).vi"("Input"=w523) -> ("Output"=w521:dbl)
              }
            }
            n294 = flat-sequence {
              tunnel: w503 -> [w520]
              tunnel: [w517] -> w502
              frame #0 {
                # "Repetition 2"
                n295 = call "Math SubVI - Simple (PCR) (DBG OFF) (INLN).vi"("Input"=w520) -> ("Output"=w518:dbl)
                n296 = call "Math SubVI - Medium (PCR) (DBG OFF) (INLN).vi"("Input"=w518) -> ("Output"=w519:dbl)
                n297 = call "Math SubVI - Complex (PCR) (DBG OFF) (INLN).vi"("Input"=w519) -> ("Output"=w517:dbl)
              }
            }
            n298 = flat-sequence {
              tunnel: w502 -> [w516]
              tunnel: [w513] -> w501
              frame #0 {
                # "Repetition 3"
                n299 = call "Math SubVI - Simple (PCR) (DBG OFF) (INLN).vi"("Input"=w516) -> ("Output"=w514:dbl)
                n300 = call "Math SubVI - Medium (PCR) (DBG OFF) (INLN).vi"("Input"=w514) -> ("Output"=w515:dbl)
                n301 = call "Math SubVI - Complex (PCR) (DBG OFF) (INLN).vi"("Input"=w515) -> ("Output"=w513:dbl)
              }
            }
            n302 = flat-sequence {
              tunnel: w501 -> [w512]
              tunnel: [w509] -> w500
              frame #0 {
                # "Repetition 4"
                n303 = call "Math SubVI - Simple (PCR) (DBG OFF) (INLN).vi"("Input"=w512) -> ("Output"=w510:dbl)
                n304 = call "Math SubVI - Medium (PCR) (DBG OFF) (INLN).vi"("Input"=w510) -> ("Output"=w511:dbl)
                n305 = call "Math SubVI - Complex (PCR) (DBG OFF) (INLN).vi"("Input"=w511) -> ("Output"=w509:dbl)
              }
            }
            n306 = flat-sequence {
              tunnel: w500 -> [w508]
              tunnel: [w505] -> w499
              frame #0 {
                # "Repetition 5"
                n307 = call "Math SubVI - Simple (PCR) (DBG OFF) (INLN).vi"("Input"=w508) -> ("Output"=w506:dbl)
                n308 = call "Math SubVI - Medium (PCR) (DBG OFF) (INLN).vi"("Input"=w506) -> ("Output"=w507:dbl)
                n309 = call "Math SubVI - Complex (PCR) (DBG OFF) (INLN).vi"("Input"=w507) -> ("Output"=w505:dbl)
              }
            }
          }
        }
        n310 = local read "Stop VI?"() -> (w472:bool)
      }
      n311 = for "Loop 8" {
        N: w42 -> [_]
        tunnel: [w414] -> w47 mode=indexing
        tunnel: [w415] -> w48
        i -> [w415]
        stop <- w416 stop-if-true
        n312 = Random Number (0-1)() -> (number: 0 to 1=w413:dbl)
        n313 = disable-structure shown="Enabled" {
          disable-tunnel: w413 -> [w422 w448]
          disable-tunnel: [w421 w443] -> w414
          frame Enabled {
            # "Case 1: Subroutines"
            n314 = flat-sequence {
              tunnel: w422 -> [w442]
              tunnel: [w439] -> w417
              frame #0 {
                # "Repetition 1"
                n315 = call "Math SubVI - Simple (PCR) (DBG OFF) (SBRTN).vi"("Input"=w442) -> ("Output"=w440:dbl)
                n316 = call "Math SubVI - Medium (PCR) (DBG OFF) (SBRTN).vi"("Input"=w440) -> ("Output"=w441:dbl)
                n317 = call "Math SubVI - Complex (PCR) (DBG OFF) (SBRTN).vi"("Input"=w441) -> ("Output"=w439:dbl)
              }
            }
            n318 = flat-sequence {
              tunnel: w417 -> [w438]
              tunnel: [w435] -> w420
              frame #0 {
                # "Repetition 2"
                n319 = call "Math SubVI - Simple (PCR) (DBG OFF) (SBRTN).vi"("Input"=w438) -> ("Output"=w436:dbl)
                n320 = call "Math SubVI - Medium (PCR) (DBG OFF) (SBRTN).vi"("Input"=w436) -> ("Output"=w437:dbl)
                n321 = call "Math SubVI - Complex (PCR) (DBG OFF) (SBRTN).vi"("Input"=w437) -> ("Output"=w435:dbl)
              }
            }
            n322 = flat-sequence {
              tunnel: w420 -> [w434]
              tunnel: [w431] -> w419
              frame #0 {
                # "Repetition 3"
                n323 = call "Math SubVI - Simple (PCR) (DBG OFF) (SBRTN).vi"("Input"=w434) -> ("Output"=w432:dbl)
                n324 = call "Math SubVI - Medium (PCR) (DBG OFF) (SBRTN).vi"("Input"=w432) -> ("Output"=w433:dbl)
                n325 = call "Math SubVI - Complex (PCR) (DBG OFF) (SBRTN).vi"("Input"=w433) -> ("Output"=w431:dbl)
              }
            }
            n326 = flat-sequence {
              tunnel: w419 -> [w430]
              tunnel: [w427] -> w418
              frame #0 {
                # "Repetition 4"
                n327 = call "Math SubVI - Simple (PCR) (DBG OFF) (SBRTN).vi"("Input"=w430) -> ("Output"=w428:dbl)
                n328 = call "Math SubVI - Medium (PCR) (DBG OFF) (SBRTN).vi"("Input"=w428) -> ("Output"=w429:dbl)
                n329 = call "Math SubVI - Complex (PCR) (DBG OFF) (SBRTN).vi"("Input"=w429) -> ("Output"=w427:dbl)
              }
            }
            n330 = flat-sequence {
              tunnel: w418 -> [w426]
              tunnel: [w423] -> w421
              frame #0 {
                # "Repetition 5"
                n331 = call "Math SubVI - Simple (PCR) (DBG OFF) (SBRTN).vi"("Input"=w426) -> ("Output"=w424:dbl)
                n332 = call "Math SubVI - Medium (PCR) (DBG OFF) (SBRTN).vi"("Input"=w424) -> ("Output"=w425:dbl)
                n333 = call "Math SubVI - Complex (PCR) (DBG OFF) (SBRTN).vi"("Input"=w425) -> ("Output"=w423:dbl)
              }
            }
          }
          frame Disabled {
            # "Case 2: Inline VIs"
            n334 = flat-sequence {
              tunnel: w448 -> [w468]
              tunnel: [w465] -> w447
              frame #0 {
                # "Repetition 1"
                n335 = call "Math SubVI - Simple (PCR) (DBG OFF) (INLN).vi"("Input"=w468) -> ("Output"=w466:dbl)
                n336 = call "Math SubVI - Medium (PCR) (DBG OFF) (INLN).vi"("Input"=w466) -> ("Output"=w467:dbl)
                n337 = call "Math SubVI - Complex (PCR) (DBG OFF) (INLN).vi"("Input"=w467) -> ("Output"=w465:dbl)
              }
            }
            n338 = flat-sequence {
              tunnel: w447 -> [w464]
              tunnel: [w461] -> w446
              frame #0 {
                # "Repetition 2"
                n339 = call "Math SubVI - Simple (PCR) (DBG OFF) (INLN).vi"("Input"=w464) -> ("Output"=w462:dbl)
                n340 = call "Math SubVI - Medium (PCR) (DBG OFF) (INLN).vi"("Input"=w462) -> ("Output"=w463:dbl)
                n341 = call "Math SubVI - Complex (PCR) (DBG OFF) (INLN).vi"("Input"=w463) -> ("Output"=w461:dbl)
              }
            }
            n342 = flat-sequence {
              tunnel: w446 -> [w460]
              tunnel: [w457] -> w445
              frame #0 {
                # "Repetition 3"
                n343 = call "Math SubVI - Simple (PCR) (DBG OFF) (INLN).vi"("Input"=w460) -> ("Output"=w458:dbl)
                n344 = call "Math SubVI - Medium (PCR) (DBG OFF) (INLN).vi"("Input"=w458) -> ("Output"=w459:dbl)
                n345 = call "Math SubVI - Complex (PCR) (DBG OFF) (INLN).vi"("Input"=w459) -> ("Output"=w457:dbl)
              }
            }
            n346 = flat-sequence {
              tunnel: w445 -> [w456]
              tunnel: [w453] -> w444
              frame #0 {
                # "Repetition 4"
                n347 = call "Math SubVI - Simple (PCR) (DBG OFF) (INLN).vi"("Input"=w456) -> ("Output"=w454:dbl)
                n348 = call "Math SubVI - Medium (PCR) (DBG OFF) (INLN).vi"("Input"=w454) -> ("Output"=w455:dbl)
                n349 = call "Math SubVI - Complex (PCR) (DBG OFF) (INLN).vi"("Input"=w455) -> ("Output"=w453:dbl)
              }
            }
            n350 = flat-sequence {
              tunnel: w444 -> [w452]
              tunnel: [w449] -> w443
              frame #0 {
                # "Repetition 5"
                n351 = call "Math SubVI - Simple (PCR) (DBG OFF) (INLN).vi"("Input"=w452) -> ("Output"=w450:dbl)
                n352 = call "Math SubVI - Medium (PCR) (DBG OFF) (INLN).vi"("Input"=w450) -> ("Output"=w451:dbl)
                n353 = call "Math SubVI - Complex (PCR) (DBG OFF) (INLN).vi"("Input"=w451) -> ("Output"=w449:dbl)
              }
            }
          }
        }
        n354 = local read "Stop VI?"() -> (w416:bool)
      }
      n355 = for "Loop 9" {
        N: w42 -> [_]
        tunnel: [w358] -> w45 mode=indexing
        tunnel: [w359] -> w46
        i -> [w359]
        stop <- w360 stop-if-true
        n356 = Random Number (0-1)() -> (number: 0 to 1=w357:dbl)
        n357 = disable-structure shown="Enabled" {
          disable-tunnel: w357 -> [w366 w392]
          disable-tunnel: [w365 w387] -> w358
          frame Enabled {
            # "Case 1: Subroutines"
            n358 = flat-sequence {
              tunnel: w366 -> [w386]
              tunnel: [w383] -> w361
              frame #0 {
                # "Repetition 1"
                n359 = call "Math SubVI - Simple (PCR) (DBG OFF) (SBRTN).vi"("Input"=w386) -> ("Output"=w384:dbl)
                n360 = call "Math SubVI - Medium (PCR) (DBG OFF) (SBRTN).vi"("Input"=w384) -> ("Output"=w385:dbl)
                n361 = call "Math SubVI - Complex (PCR) (DBG OFF) (SBRTN).vi"("Input"=w385) -> ("Output"=w383:dbl)
              }
            }
            n362 = flat-sequence {
              tunnel: w361 -> [w382]
              tunnel: [w379] -> w364
              frame #0 {
                # "Repetition 2"
                n363 = call "Math SubVI - Simple (PCR) (DBG OFF) (SBRTN).vi"("Input"=w382) -> ("Output"=w380:dbl)
                n364 = call "Math SubVI - Medium (PCR) (DBG OFF) (SBRTN).vi"("Input"=w380) -> ("Output"=w381:dbl)
                n365 = call "Math SubVI - Complex (PCR) (DBG OFF) (SBRTN).vi"("Input"=w381) -> ("Output"=w379:dbl)
              }
            }
            n366 = flat-sequence {
              tunnel: w364 -> [w378]
              tunnel: [w375] -> w363
              frame #0 {
                # "Repetition 3"
                n367 = call "Math SubVI - Simple (PCR) (DBG OFF) (SBRTN).vi"("Input"=w378) -> ("Output"=w376:dbl)
                n368 = call "Math SubVI - Medium (PCR) (DBG OFF) (SBRTN).vi"("Input"=w376) -> ("Output"=w377:dbl)
                n369 = call "Math SubVI - Complex (PCR) (DBG OFF) (SBRTN).vi"("Input"=w377) -> ("Output"=w375:dbl)
              }
            }
            n370 = flat-sequence {
              tunnel: w363 -> [w374]
              tunnel: [w371] -> w362
              frame #0 {
                # "Repetition 4"
                n371 = call "Math SubVI - Simple (PCR) (DBG OFF) (SBRTN).vi"("Input"=w374) -> ("Output"=w372:dbl)
                n372 = call "Math SubVI - Medium (PCR) (DBG OFF) (SBRTN).vi"("Input"=w372) -> ("Output"=w373:dbl)
                n373 = call "Math SubVI - Complex (PCR) (DBG OFF) (SBRTN).vi"("Input"=w373) -> ("Output"=w371:dbl)
              }
            }
            n374 = flat-sequence {
              tunnel: w362 -> [w370]
              tunnel: [w367] -> w365
              frame #0 {
                # "Repetition 5"
                n375 = call "Math SubVI - Simple (PCR) (DBG OFF) (SBRTN).vi"("Input"=w370) -> ("Output"=w368:dbl)
                n376 = call "Math SubVI - Medium (PCR) (DBG OFF) (SBRTN).vi"("Input"=w368) -> ("Output"=w369:dbl)
                n377 = call "Math SubVI - Complex (PCR) (DBG OFF) (SBRTN).vi"("Input"=w369) -> ("Output"=w367:dbl)
              }
            }
          }
          frame Disabled {
            # "Case 2: Inline VIs"
            n378 = flat-sequence {
              tunnel: w392 -> [w412]
              tunnel: [w409] -> w391
              frame #0 {
                # "Repetition 1"
                n379 = call "Math SubVI - Simple (PCR) (DBG OFF) (INLN).vi"("Input"=w412) -> ("Output"=w410:dbl)
                n380 = call "Math SubVI - Medium (PCR) (DBG OFF) (INLN).vi"("Input"=w410) -> ("Output"=w411:dbl)
                n381 = call "Math SubVI - Complex (PCR) (DBG OFF) (INLN).vi"("Input"=w411) -> ("Output"=w409:dbl)
              }
            }
            n382 = flat-sequence {
              tunnel: w391 -> [w408]
              tunnel: [w405] -> w390
              frame #0 {
                # "Repetition 2"
                n383 = call "Math SubVI - Simple (PCR) (DBG OFF) (INLN).vi"("Input"=w408) -> ("Output"=w406:dbl)
                n384 = call "Math SubVI - Medium (PCR) (DBG OFF) (INLN).vi"("Input"=w406) -> ("Output"=w407:dbl)
                n385 = call "Math SubVI - Complex (PCR) (DBG OFF) (INLN).vi"("Input"=w407) -> ("Output"=w405:dbl)
              }
            }
            n386 = flat-sequence {
              tunnel: w390 -> [w404]
              tunnel: [w401] -> w389
              frame #0 {
                # "Repetition 3"
                n387 = call "Math SubVI - Simple (PCR) (DBG OFF) (INLN).vi"("Input"=w404) -> ("Output"=w402:dbl)
                n388 = call "Math SubVI - Medium (PCR) (DBG OFF) (INLN).vi"("Input"=w402) -> ("Output"=w403:dbl)
                n389 = call "Math SubVI - Complex (PCR) (DBG OFF) (INLN).vi"("Input"=w403) -> ("Output"=w401:dbl)
              }
            }
            n390 = flat-sequence {
              tunnel: w389 -> [w400]
              tunnel: [w397] -> w388
              frame #0 {
                # "Repetition 4"
                n391 = call "Math SubVI - Simple (PCR) (DBG OFF) (INLN).vi"("Input"=w400) -> ("Output"=w398:dbl)
                n392 = call "Math SubVI - Medium (PCR) (DBG OFF) (INLN).vi"("Input"=w398) -> ("Output"=w399:dbl)
                n393 = call "Math SubVI - Complex (PCR) (DBG OFF) (INLN).vi"("Input"=w399) -> ("Output"=w397:dbl)
              }
            }
            n394 = flat-sequence {
              tunnel: w388 -> [w396]
              tunnel: [w393] -> w387
              frame #0 {
                # "Repetition 5"
                n395 = call "Math SubVI - Simple (PCR) (DBG OFF) (INLN).vi"("Input"=w396) -> ("Output"=w394:dbl)
                n396 = call "Math SubVI - Medium (PCR) (DBG OFF) (INLN).vi"("Input"=w394) -> ("Output"=w395:dbl)
                n397 = call "Math SubVI - Complex (PCR) (DBG OFF) (INLN).vi"("Input"=w395) -> ("Output"=w393:dbl)
              }
            }
          }
        }
        n398 = local read "Stop VI?"() -> (w360:bool)
      }
      n399 = for "Loop 10" {
        N: w42 -> [_]
        tunnel: [w302] -> w43 mode=indexing
        tunnel: [w303] -> w44
        i -> [w303]
        stop <- w304 stop-if-true
        n400 = Random Number (0-1)() -> (number: 0 to 1=w301:dbl)
        n401 = disable-structure shown="Enabled" {
          disable-tunnel: w301 -> [w310 w336]
          disable-tunnel: [w309 w331] -> w302
          frame Enabled {
            # "Case 1: Subroutines"
            n402 = flat-sequence {
              tunnel: w310 -> [w330]
              tunnel: [w327] -> w305
              frame #0 {
                # "Repetition 1"
                n403 = call "Math SubVI - Simple (PCR) (DBG OFF) (SBRTN).vi"("Input"=w330) -> ("Output"=w328:dbl)
                n404 = call "Math SubVI - Medium (PCR) (DBG OFF) (SBRTN).vi"("Input"=w328) -> ("Output"=w329:dbl)
                n405 = call "Math SubVI - Complex (PCR) (DBG OFF) (SBRTN).vi"("Input"=w329) -> ("Output"=w327:dbl)
              }
            }
            n406 = flat-sequence {
              tunnel: w305 -> [w326]
              tunnel: [w323] -> w308
              frame #0 {
                # "Repetition 2"
                n407 = call "Math SubVI - Simple (PCR) (DBG OFF) (SBRTN).vi"("Input"=w326) -> ("Output"=w324:dbl)
                n408 = call "Math SubVI - Medium (PCR) (DBG OFF) (SBRTN).vi"("Input"=w324) -> ("Output"=w325:dbl)
                n409 = call "Math SubVI - Complex (PCR) (DBG OFF) (SBRTN).vi"("Input"=w325) -> ("Output"=w323:dbl)
              }
            }
            n410 = flat-sequence {
              tunnel: w308 -> [w322]
              tunnel: [w319] -> w307
              frame #0 {
                # "Repetition 3"
                n411 = call "Math SubVI - Simple (PCR) (DBG OFF) (SBRTN).vi"("Input"=w322) -> ("Output"=w320:dbl)
                n412 = call "Math SubVI - Medium (PCR) (DBG OFF) (SBRTN).vi"("Input"=w320) -> ("Output"=w321:dbl)
                n413 = call "Math SubVI - Complex (PCR) (DBG OFF) (SBRTN).vi"("Input"=w321) -> ("Output"=w319:dbl)
              }
            }
            n414 = flat-sequence {
              tunnel: w307 -> [w318]
              tunnel: [w315] -> w306
              frame #0 {
                # "Repetition 4"
                n415 = call "Math SubVI - Simple (PCR) (DBG OFF) (SBRTN).vi"("Input"=w318) -> ("Output"=w316:dbl)
                n416 = call "Math SubVI - Medium (PCR) (DBG OFF) (SBRTN).vi"("Input"=w316) -> ("Output"=w317:dbl)
                n417 = call "Math SubVI - Complex (PCR) (DBG OFF) (SBRTN).vi"("Input"=w317) -> ("Output"=w315:dbl)
              }
            }
            n418 = flat-sequence {
              tunnel: w306 -> [w314]
              tunnel: [w311] -> w309
              frame #0 {
                # "Repetition 5"
                n419 = call "Math SubVI - Simple (PCR) (DBG OFF) (SBRTN).vi"("Input"=w314) -> ("Output"=w312:dbl)
                n420 = call "Math SubVI - Medium (PCR) (DBG OFF) (SBRTN).vi"("Input"=w312) -> ("Output"=w313:dbl)
                n421 = call "Math SubVI - Complex (PCR) (DBG OFF) (SBRTN).vi"("Input"=w313) -> ("Output"=w311:dbl)
              }
            }
          }
          frame Disabled {
            # "Case 2: Inline VIs"
            n422 = flat-sequence {
              tunnel: w336 -> [w356]
              tunnel: [w353] -> w335
              frame #0 {
                # "Repetition 1"
                n423 = call "Math SubVI - Simple (PCR) (DBG OFF) (INLN).vi"("Input"=w356) -> ("Output"=w354:dbl)
                n424 = call "Math SubVI - Medium (PCR) (DBG OFF) (INLN).vi"("Input"=w354) -> ("Output"=w355:dbl)
                n425 = call "Math SubVI - Complex (PCR) (DBG OFF) (INLN).vi"("Input"=w355) -> ("Output"=w353:dbl)
              }
            }
            n426 = flat-sequence {
              tunnel: w335 -> [w352]
              tunnel: [w349] -> w334
              frame #0 {
                # "Repetition 2"
                n427 = call "Math SubVI - Simple (PCR) (DBG OFF) (INLN).vi"("Input"=w352) -> ("Output"=w350:dbl)
                n428 = call "Math SubVI - Medium (PCR) (DBG OFF) (INLN).vi"("Input"=w350) -> ("Output"=w351:dbl)
                n429 = call "Math SubVI - Complex (PCR) (DBG OFF) (INLN).vi"("Input"=w351) -> ("Output"=w349:dbl)
              }
            }
            n430 = flat-sequence {
              tunnel: w334 -> [w348]
              tunnel: [w345] -> w333
              frame #0 {
                # "Repetition 3"
                n431 = call "Math SubVI - Simple (PCR) (DBG OFF) (INLN).vi"("Input"=w348) -> ("Output"=w346:dbl)
                n432 = call "Math SubVI - Medium (PCR) (DBG OFF) (INLN).vi"("Input"=w346) -> ("Output"=w347:dbl)
                n433 = call "Math SubVI - Complex (PCR) (DBG OFF) (INLN).vi"("Input"=w347) -> ("Output"=w345:dbl)
              }
            }
            n434 = flat-sequence {
              tunnel: w333 -> [w344]
              tunnel: [w341] -> w332
              frame #0 {
                # "Repetition 4"
                n435 = call "Math SubVI - Simple (PCR) (DBG OFF) (INLN).vi"("Input"=w344) -> ("Output"=w342:dbl)
                n436 = call "Math SubVI - Medium (PCR) (DBG OFF) (INLN).vi"("Input"=w342) -> ("Output"=w343:dbl)
                n437 = call "Math SubVI - Complex (PCR) (DBG OFF) (INLN).vi"("Input"=w343) -> ("Output"=w341:dbl)
              }
            }
            n438 = flat-sequence {
              tunnel: w332 -> [w340]
              tunnel: [w337] -> w331
              frame #0 {
                # "Repetition 5"
                n439 = call "Math SubVI - Simple (PCR) (DBG OFF) (INLN).vi"("Input"=w340) -> ("Output"=w338:dbl)
                n440 = call "Math SubVI - Medium (PCR) (DBG OFF) (INLN).vi"("Input"=w338) -> ("Output"=w339:dbl)
                n441 = call "Math SubVI - Complex (PCR) (DBG OFF) (INLN).vi"("Input"=w339) -> ("Output"=w337:dbl)
              }
            }
          }
        }
        n442 = local read "Stop VI?"() -> (w304:bool)
      }
      n443 = for "Loop 11" {
        N: w42 -> [_]
        tunnel: [w244] -> w41 mode=indexing
        tunnel: [w245] -> w40
        i -> [w245]
        stop <- w246 stop-if-true
        n444 = Random Number (0-1)() -> (number: 0 to 1=w243:dbl)
        n445 = disable-structure shown="Enabled" {
          disable-tunnel: w243 -> [w252 w278]
          disable-tunnel: [w251 w273] -> w244
          frame Enabled {
            # "Case 1: Subroutines"
            n446 = flat-sequence {
              tunnel: w252 -> [w272]
              tunnel: [w269] -> w247
              frame #0 {
                # "Repetition 1"
                n447 = call "Math SubVI - Simple (PCR) (DBG OFF) (SBRTN).vi"("Input"=w272) -> ("Output"=w270:dbl)
                n448 = call "Math SubVI - Medium (PCR) (DBG OFF) (SBRTN).vi"("Input"=w270) -> ("Output"=w271:dbl)
                n449 = call "Math SubVI - Complex (PCR) (DBG OFF) (SBRTN).vi"("Input"=w271) -> ("Output"=w269:dbl)
              }
            }
            n450 = flat-sequence {
              tunnel: w247 -> [w268]
              tunnel: [w265] -> w250
              frame #0 {
                # "Repetition 2"
                n451 = call "Math SubVI - Simple (PCR) (DBG OFF) (SBRTN).vi"("Input"=w268) -> ("Output"=w266:dbl)
                n452 = call "Math SubVI - Medium (PCR) (DBG OFF) (SBRTN).vi"("Input"=w266) -> ("Output"=w267:dbl)
                n453 = call "Math SubVI - Complex (PCR) (DBG OFF) (SBRTN).vi"("Input"=w267) -> ("Output"=w265:dbl)
              }
            }
            n454 = flat-sequence {
              tunnel: w250 -> [w264]
              tunnel: [w261] -> w249
              frame #0 {
                # "Repetition 3"
                n455 = call "Math SubVI - Simple (PCR) (DBG OFF) (SBRTN).vi"("Input"=w264) -> ("Output"=w262:dbl)
                n456 = call "Math SubVI - Medium (PCR) (DBG OFF) (SBRTN).vi"("Input"=w262) -> ("Output"=w263:dbl)
                n457 = call "Math SubVI - Complex (PCR) (DBG OFF) (SBRTN).vi"("Input"=w263) -> ("Output"=w261:dbl)
              }
            }
            n458 = flat-sequence {
              tunnel: w249 -> [w260]
              tunnel: [w257] -> w248
              frame #0 {
                # "Repetition 4"
                n459 = call "Math SubVI - Simple (PCR) (DBG OFF) (SBRTN).vi"("Input"=w260) -> ("Output"=w258:dbl)
                n460 = call "Math SubVI - Medium (PCR) (DBG OFF) (SBRTN).vi"("Input"=w258) -> ("Output"=w259:dbl)
                n461 = call "Math SubVI - Complex (PCR) (DBG OFF) (SBRTN).vi"("Input"=w259) -> ("Output"=w257:dbl)
              }
            }
            n462 = flat-sequence {
              tunnel: w248 -> [w256]
              tunnel: [w253] -> w251
              frame #0 {
                # "Repetition 5"
                n463 = call "Math SubVI - Simple (PCR) (DBG OFF) (SBRTN).vi"("Input"=w256) -> ("Output"=w254:dbl)
                n464 = call "Math SubVI - Medium (PCR) (DBG OFF) (SBRTN).vi"("Input"=w254) -> ("Output"=w255:dbl)
                n465 = call "Math SubVI - Complex (PCR) (DBG OFF) (SBRTN).vi"("Input"=w255) -> ("Output"=w253:dbl)
              }
            }
          }
          frame Disabled {
            # "Case 2: Inline VIs"
            n466 = flat-sequence {
              tunnel: w278 -> [w298]
              tunnel: [w295] -> w277
              frame #0 {
                # "Repetition 1"
                n467 = call "Math SubVI - Simple (PCR) (DBG OFF) (INLN).vi"("Input"=w298) -> ("Output"=w296:dbl)
                n468 = call "Math SubVI - Medium (PCR) (DBG OFF) (INLN).vi"("Input"=w296) -> ("Output"=w297:dbl)
                n469 = call "Math SubVI - Complex (PCR) (DBG OFF) (INLN).vi"("Input"=w297) -> ("Output"=w295:dbl)
              }
            }
            n470 = flat-sequence {
              tunnel: w277 -> [w294]
              tunnel: [w291] -> w276
              frame #0 {
                # "Repetition 2"
                n471 = call "Math SubVI - Simple (PCR) (DBG OFF) (INLN).vi"("Input"=w294) -> ("Output"=w292:dbl)
                n472 = call "Math SubVI - Medium (PCR) (DBG OFF) (INLN).vi"("Input"=w292) -> ("Output"=w293:dbl)
                n473 = call "Math SubVI - Complex (PCR) (DBG OFF) (INLN).vi"("Input"=w293) -> ("Output"=w291:dbl)
              }
            }
            n474 = flat-sequence {
              tunnel: w276 -> [w290]
              tunnel: [w287] -> w275
              frame #0 {
                # "Repetition 3"
                n475 = call "Math SubVI - Simple (PCR) (DBG OFF) (INLN).vi"("Input"=w290) -> ("Output"=w288:dbl)
                n476 = call "Math SubVI - Medium (PCR) (DBG OFF) (INLN).vi"("Input"=w288) -> ("Output"=w289:dbl)
                n477 = call "Math SubVI - Complex (PCR) (DBG OFF) (INLN).vi"("Input"=w289) -> ("Output"=w287:dbl)
              }
            }
            n478 = flat-sequence {
              tunnel: w275 -> [w286]
              tunnel: [w283] -> w274
              frame #0 {
                # "Repetition 4"
                n479 = call "Math SubVI - Simple (PCR) (DBG OFF) (INLN).vi"("Input"=w286) -> ("Output"=w284:dbl)
                n480 = call "Math SubVI - Medium (PCR) (DBG OFF) (INLN).vi"("Input"=w284) -> ("Output"=w285:dbl)
                n481 = call "Math SubVI - Complex (PCR) (DBG OFF) (INLN).vi"("Input"=w285) -> ("Output"=w283:dbl)
              }
            }
            n482 = flat-sequence {
              tunnel: w274 -> [w282]
              tunnel: [w279] -> w273
              frame #0 {
                # "Repetition 5"
                n483 = call "Math SubVI - Simple (PCR) (DBG OFF) (INLN).vi"("Input"=w282) -> ("Output"=w280:dbl)
                n484 = call "Math SubVI - Medium (PCR) (DBG OFF) (INLN).vi"("Input"=w280) -> ("Output"=w281:dbl)
                n485 = call "Math SubVI - Complex (PCR) (DBG OFF) (INLN).vi"("Input"=w281) -> ("Output"=w279:dbl)
              }
            }
          }
        }
        n486 = local read "Stop VI?"() -> (w246:bool)
      }
      n487 = for "Loop 12" {
        N: w42 -> [_]
        tunnel: [w188] -> w38 mode=indexing
        tunnel: [w189] -> w37
        i -> [w189]
        stop <- w190 stop-if-true
        n488 = Random Number (0-1)() -> (number: 0 to 1=w187:dbl)
        n489 = disable-structure shown="Enabled" {
          disable-tunnel: w187 -> [w196 w222]
          disable-tunnel: [w195 w217] -> w188
          frame Enabled {
            # "Case 1: Subroutines"
            n490 = flat-sequence {
              tunnel: w196 -> [w216]
              tunnel: [w213] -> w191
              frame #0 {
                # "Repetition 1"
                n491 = call "Math SubVI - Simple (PCR) (DBG OFF) (SBRTN).vi"("Input"=w216) -> ("Output"=w214:dbl)
                n492 = call "Math SubVI - Medium (PCR) (DBG OFF) (SBRTN).vi"("Input"=w214) -> ("Output"=w215:dbl)
                n493 = call "Math SubVI - Complex (PCR) (DBG OFF) (SBRTN).vi"("Input"=w215) -> ("Output"=w213:dbl)
              }
            }
            n494 = flat-sequence {
              tunnel: w191 -> [w212]
              tunnel: [w209] -> w194
              frame #0 {
                # "Repetition 2"
                n495 = call "Math SubVI - Simple (PCR) (DBG OFF) (SBRTN).vi"("Input"=w212) -> ("Output"=w210:dbl)
                n496 = call "Math SubVI - Medium (PCR) (DBG OFF) (SBRTN).vi"("Input"=w210) -> ("Output"=w211:dbl)
                n497 = call "Math SubVI - Complex (PCR) (DBG OFF) (SBRTN).vi"("Input"=w211) -> ("Output"=w209:dbl)
              }
            }
            n498 = flat-sequence {
              tunnel: w194 -> [w208]
              tunnel: [w205] -> w193
              frame #0 {
                # "Repetition 3"
                n499 = call "Math SubVI - Simple (PCR) (DBG OFF) (SBRTN).vi"("Input"=w208) -> ("Output"=w206:dbl)
                n500 = call "Math SubVI - Medium (PCR) (DBG OFF) (SBRTN).vi"("Input"=w206) -> ("Output"=w207:dbl)
                n501 = call "Math SubVI - Complex (PCR) (DBG OFF) (SBRTN).vi"("Input"=w207) -> ("Output"=w205:dbl)
              }
            }
            n502 = flat-sequence {
              tunnel: w193 -> [w204]
              tunnel: [w201] -> w192
              frame #0 {
                # "Repetition 4"
                n503 = call "Math SubVI - Simple (PCR) (DBG OFF) (SBRTN).vi"("Input"=w204) -> ("Output"=w202:dbl)
                n504 = call "Math SubVI - Medium (PCR) (DBG OFF) (SBRTN).vi"("Input"=w202) -> ("Output"=w203:dbl)
                n505 = call "Math SubVI - Complex (PCR) (DBG OFF) (SBRTN).vi"("Input"=w203) -> ("Output"=w201:dbl)
              }
            }
            n506 = flat-sequence {
              tunnel: w192 -> [w200]
              tunnel: [w197] -> w195
              frame #0 {
                # "Repetition 5"
                n507 = call "Math SubVI - Simple (PCR) (DBG OFF) (SBRTN).vi"("Input"=w200) -> ("Output"=w198:dbl)
                n508 = call "Math SubVI - Medium (PCR) (DBG OFF) (SBRTN).vi"("Input"=w198) -> ("Output"=w199:dbl)
                n509 = call "Math SubVI - Complex (PCR) (DBG OFF) (SBRTN).vi"("Input"=w199) -> ("Output"=w197:dbl)
              }
            }
          }
          frame Disabled {
            # "Case 2: Inline VIs"
            n510 = flat-sequence {
              tunnel: w222 -> [w242]
              tunnel: [w239] -> w221
              frame #0 {
                # "Repetition 1"
                n511 = call "Math SubVI - Simple (PCR) (DBG OFF) (INLN).vi"("Input"=w242) -> ("Output"=w240:dbl)
                n512 = call "Math SubVI - Medium (PCR) (DBG OFF) (INLN).vi"("Input"=w240) -> ("Output"=w241:dbl)
                n513 = call "Math SubVI - Complex (PCR) (DBG OFF) (INLN).vi"("Input"=w241) -> ("Output"=w239:dbl)
              }
            }
            n514 = flat-sequence {
              tunnel: w221 -> [w238]
              tunnel: [w235] -> w220
              frame #0 {
                # "Repetition 2"
                n515 = call "Math SubVI - Simple (PCR) (DBG OFF) (INLN).vi"("Input"=w238) -> ("Output"=w236:dbl)
                n516 = call "Math SubVI - Medium (PCR) (DBG OFF) (INLN).vi"("Input"=w236) -> ("Output"=w237:dbl)
                n517 = call "Math SubVI - Complex (PCR) (DBG OFF) (INLN).vi"("Input"=w237) -> ("Output"=w235:dbl)
              }
            }
            n518 = flat-sequence {
              tunnel: w220 -> [w234]
              tunnel: [w231] -> w219
              frame #0 {
                # "Repetition 3"
                n519 = call "Math SubVI - Simple (PCR) (DBG OFF) (INLN).vi"("Input"=w234) -> ("Output"=w232:dbl)
                n520 = call "Math SubVI - Medium (PCR) (DBG OFF) (INLN).vi"("Input"=w232) -> ("Output"=w233:dbl)
                n521 = call "Math SubVI - Complex (PCR) (DBG OFF) (INLN).vi"("Input"=w233) -> ("Output"=w231:dbl)
              }
            }
            n522 = flat-sequence {
              tunnel: w219 -> [w230]
              tunnel: [w227] -> w218
              frame #0 {
                # "Repetition 4"
                n523 = call "Math SubVI - Simple (PCR) (DBG OFF) (INLN).vi"("Input"=w230) -> ("Output"=w228:dbl)
                n524 = call "Math SubVI - Medium (PCR) (DBG OFF) (INLN).vi"("Input"=w228) -> ("Output"=w229:dbl)
                n525 = call "Math SubVI - Complex (PCR) (DBG OFF) (INLN).vi"("Input"=w229) -> ("Output"=w227:dbl)
              }
            }
            n526 = flat-sequence {
              tunnel: w218 -> [w226]
              tunnel: [w223] -> w217
              frame #0 {
                # "Repetition 5"
                n527 = call "Math SubVI - Simple (PCR) (DBG OFF) (INLN).vi"("Input"=w226) -> ("Output"=w224:dbl)
                n528 = call "Math SubVI - Medium (PCR) (DBG OFF) (INLN).vi"("Input"=w224) -> ("Output"=w225:dbl)
                n529 = call "Math SubVI - Complex (PCR) (DBG OFF) (INLN).vi"("Input"=w225) -> ("Output"=w223:dbl)
              }
            }
          }
        }
        n530 = local read "Stop VI?"() -> (w190:bool)
      }
      n531 = for "Loop 13" {
        N: w42 -> [_]
        tunnel: [w132] -> w36 mode=indexing
        tunnel: [w133] -> w35
        i -> [w133]
        stop <- w134 stop-if-true
        n532 = Random Number (0-1)() -> (number: 0 to 1=w131:dbl)
        n533 = disable-structure shown="Enabled" {
          disable-tunnel: w131 -> [w140 w166]
          disable-tunnel: [w139 w161] -> w132
          frame Enabled {
            # "Case 1: Subroutines"
            n534 = flat-sequence {
              tunnel: w140 -> [w160]
              tunnel: [w157] -> w135
              frame #0 {
                # "Repetition 1"
                n535 = call "Math SubVI - Simple (PCR) (DBG OFF) (SBRTN).vi"("Input"=w160) -> ("Output"=w158:dbl)
                n536 = call "Math SubVI - Medium (PCR) (DBG OFF) (SBRTN).vi"("Input"=w158) -> ("Output"=w159:dbl)
                n537 = call "Math SubVI - Complex (PCR) (DBG OFF) (SBRTN).vi"("Input"=w159) -> ("Output"=w157:dbl)
              }
            }
            n538 = flat-sequence {
              tunnel: w135 -> [w156]
              tunnel: [w153] -> w138
              frame #0 {
                # "Repetition 2"
                n539 = call "Math SubVI - Simple (PCR) (DBG OFF) (SBRTN).vi"("Input"=w156) -> ("Output"=w154:dbl)
                n540 = call "Math SubVI - Medium (PCR) (DBG OFF) (SBRTN).vi"("Input"=w154) -> ("Output"=w155:dbl)
                n541 = call "Math SubVI - Complex (PCR) (DBG OFF) (SBRTN).vi"("Input"=w155) -> ("Output"=w153:dbl)
              }
            }
            n542 = flat-sequence {
              tunnel: w138 -> [w152]
              tunnel: [w149] -> w137
              frame #0 {
                # "Repetition 3"
                n543 = call "Math SubVI - Simple (PCR) (DBG OFF) (SBRTN).vi"("Input"=w152) -> ("Output"=w150:dbl)
                n544 = call "Math SubVI - Medium (PCR) (DBG OFF) (SBRTN).vi"("Input"=w150) -> ("Output"=w151:dbl)
                n545 = call "Math SubVI - Complex (PCR) (DBG OFF) (SBRTN).vi"("Input"=w151) -> ("Output"=w149:dbl)
              }
            }
            n546 = flat-sequence {
              tunnel: w137 -> [w148]
              tunnel: [w145] -> w136
              frame #0 {
                # "Repetition 4"
                n547 = call "Math SubVI - Simple (PCR) (DBG OFF) (SBRTN).vi"("Input"=w148) -> ("Output"=w146:dbl)
                n548 = call "Math SubVI - Medium (PCR) (DBG OFF) (SBRTN).vi"("Input"=w146) -> ("Output"=w147:dbl)
                n549 = call "Math SubVI - Complex (PCR) (DBG OFF) (SBRTN).vi"("Input"=w147) -> ("Output"=w145:dbl)
              }
            }
            n550 = flat-sequence {
              tunnel: w136 -> [w144]
              tunnel: [w141] -> w139
              frame #0 {
                # "Repetition 5"
                n551 = call "Math SubVI - Simple (PCR) (DBG OFF) (SBRTN).vi"("Input"=w144) -> ("Output"=w142:dbl)
                n552 = call "Math SubVI - Medium (PCR) (DBG OFF) (SBRTN).vi"("Input"=w142) -> ("Output"=w143:dbl)
                n553 = call "Math SubVI - Complex (PCR) (DBG OFF) (SBRTN).vi"("Input"=w143) -> ("Output"=w141:dbl)
              }
            }
          }
          frame Disabled {
            # "Case 2: Inline VIs"
            n554 = flat-sequence {
              tunnel: w166 -> [w186]
              tunnel: [w183] -> w165
              frame #0 {
                # "Repetition 1"
                n555 = call "Math SubVI - Simple (PCR) (DBG OFF) (INLN).vi"("Input"=w186) -> ("Output"=w184:dbl)
                n556 = call "Math SubVI - Medium (PCR) (DBG OFF) (INLN).vi"("Input"=w184) -> ("Output"=w185:dbl)
                n557 = call "Math SubVI - Complex (PCR) (DBG OFF) (INLN).vi"("Input"=w185) -> ("Output"=w183:dbl)
              }
            }
            n558 = flat-sequence {
              tunnel: w165 -> [w182]
              tunnel: [w179] -> w164
              frame #0 {
                # "Repetition 2"
                n559 = call "Math SubVI - Simple (PCR) (DBG OFF) (INLN).vi"("Input"=w182) -> ("Output"=w180:dbl)
                n560 = call "Math SubVI - Medium (PCR) (DBG OFF) (INLN).vi"("Input"=w180) -> ("Output"=w181:dbl)
                n561 = call "Math SubVI - Complex (PCR) (DBG OFF) (INLN).vi"("Input"=w181) -> ("Output"=w179:dbl)
              }
            }
            n562 = flat-sequence {
              tunnel: w164 -> [w178]
              tunnel: [w175] -> w163
              frame #0 {
                # "Repetition 3"
                n563 = call "Math SubVI - Simple (PCR) (DBG OFF) (INLN).vi"("Input"=w178) -> ("Output"=w176:dbl)
                n564 = call "Math SubVI - Medium (PCR) (DBG OFF) (INLN).vi"("Input"=w176) -> ("Output"=w177:dbl)
                n565 = call "Math SubVI - Complex (PCR) (DBG OFF) (INLN).vi"("Input"=w177) -> ("Output"=w175:dbl)
              }
            }
            n566 = flat-sequence {
              tunnel: w163 -> [w174]
              tunnel: [w171] -> w162
              frame #0 {
                # "Repetition 4"
                n567 = call "Math SubVI - Simple (PCR) (DBG OFF) (INLN).vi"("Input"=w174) -> ("Output"=w172:dbl)
                n568 = call "Math SubVI - Medium (PCR) (DBG OFF) (INLN).vi"("Input"=w172) -> ("Output"=w173:dbl)
                n569 = call "Math SubVI - Complex (PCR) (DBG OFF) (INLN).vi"("Input"=w173) -> ("Output"=w171:dbl)
              }
            }
            n570 = flat-sequence {
              tunnel: w162 -> [w170]
              tunnel: [w167] -> w161
              frame #0 {
                # "Repetition 5"
                n571 = call "Math SubVI - Simple (PCR) (DBG OFF) (INLN).vi"("Input"=w170) -> ("Output"=w168:dbl)
                n572 = call "Math SubVI - Medium (PCR) (DBG OFF) (INLN).vi"("Input"=w168) -> ("Output"=w169:dbl)
                n573 = call "Math SubVI - Complex (PCR) (DBG OFF) (INLN).vi"("Input"=w169) -> ("Output"=w167:dbl)
              }
            }
          }
        }
        n574 = local read "Stop VI?"() -> (w134:bool)
      }
      n575 = for "Loop 14" {
        N: w42 -> [_]
        tunnel: [w76] -> w34 mode=indexing
        tunnel: [w77] -> w33
        i -> [w77]
        stop <- w78 stop-if-true
        n576 = Random Number (0-1)() -> (number: 0 to 1=w75:dbl)
        n577 = disable-structure shown="Enabled" {
          disable-tunnel: w75 -> [w84 w110]
          disable-tunnel: [w83 w105] -> w76
          frame Enabled {
            # "Case 1: Subroutines"
            n578 = flat-sequence {
              tunnel: w84 -> [w104]
              tunnel: [w101] -> w79
              frame #0 {
                # "Repetition 1"
                n579 = call "Math SubVI - Simple (PCR) (DBG OFF) (SBRTN).vi"("Input"=w104) -> ("Output"=w102:dbl)
                n580 = call "Math SubVI - Medium (PCR) (DBG OFF) (SBRTN).vi"("Input"=w102) -> ("Output"=w103:dbl)
                n581 = call "Math SubVI - Complex (PCR) (DBG OFF) (SBRTN).vi"("Input"=w103) -> ("Output"=w101:dbl)
              }
            }
            n582 = flat-sequence {
              tunnel: w79 -> [w100]
              tunnel: [w97] -> w82
              frame #0 {
                # "Repetition 2"
                n583 = call "Math SubVI - Simple (PCR) (DBG OFF) (SBRTN).vi"("Input"=w100) -> ("Output"=w98:dbl)
                n584 = call "Math SubVI - Medium (PCR) (DBG OFF) (SBRTN).vi"("Input"=w98) -> ("Output"=w99:dbl)
                n585 = call "Math SubVI - Complex (PCR) (DBG OFF) (SBRTN).vi"("Input"=w99) -> ("Output"=w97:dbl)
              }
            }
            n586 = flat-sequence {
              tunnel: w82 -> [w96]
              tunnel: [w93] -> w81
              frame #0 {
                # "Repetition 3"
                n587 = call "Math SubVI - Simple (PCR) (DBG OFF) (SBRTN).vi"("Input"=w96) -> ("Output"=w94:dbl)
                n588 = call "Math SubVI - Medium (PCR) (DBG OFF) (SBRTN).vi"("Input"=w94) -> ("Output"=w95:dbl)
                n589 = call "Math SubVI - Complex (PCR) (DBG OFF) (SBRTN).vi"("Input"=w95) -> ("Output"=w93:dbl)
              }
            }
            n590 = flat-sequence {
              tunnel: w81 -> [w92]
              tunnel: [w89] -> w80
              frame #0 {
                # "Repetition 4"
                n591 = call "Math SubVI - Simple (PCR) (DBG OFF) (SBRTN).vi"("Input"=w92) -> ("Output"=w90:dbl)
                n592 = call "Math SubVI - Medium (PCR) (DBG OFF) (SBRTN).vi"("Input"=w90) -> ("Output"=w91:dbl)
                n593 = call "Math SubVI - Complex (PCR) (DBG OFF) (SBRTN).vi"("Input"=w91) -> ("Output"=w89:dbl)
              }
            }
            n594 = flat-sequence {
              tunnel: w80 -> [w88]
              tunnel: [w85] -> w83
              frame #0 {
                # "Repetition 5"
                n595 = call "Math SubVI - Simple (PCR) (DBG OFF) (SBRTN).vi"("Input"=w88) -> ("Output"=w86:dbl)
                n596 = call "Math SubVI - Medium (PCR) (DBG OFF) (SBRTN).vi"("Input"=w86) -> ("Output"=w87:dbl)
                n597 = call "Math SubVI - Complex (PCR) (DBG OFF) (SBRTN).vi"("Input"=w87) -> ("Output"=w85:dbl)
              }
            }
          }
          frame Disabled {
            # "Case 2: Inline VIs"
            n598 = flat-sequence {
              tunnel: w110 -> [w130]
              tunnel: [w127] -> w109
              frame #0 {
                # "Repetition 1"
                n599 = call "Math SubVI - Simple (PCR) (DBG OFF) (INLN).vi"("Input"=w130) -> ("Output"=w128:dbl)
                n600 = call "Math SubVI - Medium (PCR) (DBG OFF) (INLN).vi"("Input"=w128) -> ("Output"=w129:dbl)
                n601 = call "Math SubVI - Complex (PCR) (DBG OFF) (INLN).vi"("Input"=w129) -> ("Output"=w127:dbl)
              }
            }
            n602 = flat-sequence {
              tunnel: w109 -> [w126]
              tunnel: [w123] -> w108
              frame #0 {
                # "Repetition 2"
                n603 = call "Math SubVI - Simple (PCR) (DBG OFF) (INLN).vi"("Input"=w126) -> ("Output"=w124:dbl)
                n604 = call "Math SubVI - Medium (PCR) (DBG OFF) (INLN).vi"("Input"=w124) -> ("Output"=w125:dbl)
                n605 = call "Math SubVI - Complex (PCR) (DBG OFF) (INLN).vi"("Input"=w125) -> ("Output"=w123:dbl)
              }
            }
            n606 = flat-sequence {
              tunnel: w108 -> [w122]
              tunnel: [w119] -> w107
              frame #0 {
                # "Repetition 3"
                n607 = call "Math SubVI - Simple (PCR) (DBG OFF) (INLN).vi"("Input"=w122) -> ("Output"=w120:dbl)
                n608 = call "Math SubVI - Medium (PCR) (DBG OFF) (INLN).vi"("Input"=w120) -> ("Output"=w121:dbl)
                n609 = call "Math SubVI - Complex (PCR) (DBG OFF) (INLN).vi"("Input"=w121) -> ("Output"=w119:dbl)
              }
            }
            n610 = flat-sequence {
              tunnel: w107 -> [w118]
              tunnel: [w115] -> w106
              frame #0 {
                # "Repetition 4"
                n611 = call "Math SubVI - Simple (PCR) (DBG OFF) (INLN).vi"("Input"=w118) -> ("Output"=w116:dbl)
                n612 = call "Math SubVI - Medium (PCR) (DBG OFF) (INLN).vi"("Input"=w116) -> ("Output"=w117:dbl)
                n613 = call "Math SubVI - Complex (PCR) (DBG OFF) (INLN).vi"("Input"=w117) -> ("Output"=w115:dbl)
              }
            }
            n614 = flat-sequence {
              tunnel: w106 -> [w114]
              tunnel: [w111] -> w105
              frame #0 {
                # "Repetition 5"
                n615 = call "Math SubVI - Simple (PCR) (DBG OFF) (INLN).vi"("Input"=w114) -> ("Output"=w112:dbl)
                n616 = call "Math SubVI - Medium (PCR) (DBG OFF) (INLN).vi"("Input"=w112) -> ("Output"=w113:dbl)
                n617 = call "Math SubVI - Complex (PCR) (DBG OFF) (INLN).vi"("Input"=w113) -> ("Output"=w111:dbl)
              }
            }
          }
        }
        n618 = local read "Stop VI?"() -> (w78:bool)
      }
      n619 = call <vilib>:"High Resolution Polling Wait.vi"("seconds to wait"=w74) -> ("error out"=w73:errorcluster)  [unwired: 10 in]
      n620 = flat-sequence {
        tunnel: w73 -> [w299]
        frame #0 {
          n621 = call <vilib>:"Clear Errors.vi"("error in (no error)"=w299) -> ()  [unwired: 5 in, 2 out]
          "Stop VI?" <- TRUE
        }
      }
      n622 = Increment(x=w53) -> (x+1=w66:i32)
      n623 = Increment(x=w51) -> (x+1=w61:i32)
      n624 = Increment(x=w49) -> (x+1=w62:i32)
      n625 = Increment(x=w48) -> (x+1=w63:i32)
      n626 = Increment(x=w46) -> (x+1=w64:i32)
      n627 = Increment(x=w44) -> (x+1=w65:i32)
      n628 = Increment(x=w40) -> (x+1=w39:i32)
      n629 = Increment(x=w37) -> (x+1=w32:i32)
      n630 = Increment(x=w35) -> (x+1=w31:i32)
      n631 = Increment(x=w33) -> (x+1=w30:i32)
      n632 = Increment(x=w71) -> (x+1=w70:i32)
      n633 = Increment(x=w59) -> (x+1=w69:i32)
      n634 = Increment(x=w57) -> (x+1=w68:i32)
      n635 = Increment(x=w55) -> (x+1=w67:i32)
    }
    frame #2 {
      n636 = Build Array(w893, w892, w888, w887, w879, w878, w877, w876, w875, w874, w864, w863, w862, w861) -> (w873:i32[])
      n637 = for {
        tunnel: w873 -> [w899] mode=indexing
        tunnel: [w898] -> w872 mode=indexing
        n638 = Number To Decimal String(number=w899) -> (decimal integer string=w898:string)  [unwired: 1 in]
      }
      n639 = To Double Precision Float(number=w873) -> (double precision float=w886:dbl[])
      n640 = call-poly <vilib>:"Mean.vi"("X"=w886) -> ("mean"=w891:dbl)  [unwired: 1 out]
      "Avg. No. Of Iterations Executed - All Loops" <- w891
      n641 = disable-structure shown="Enabled" {
        disable-tunnel: w891 -> [w897 _]
        frame Disabled {
          n642 = call "Copy Result To Clipboard.vi"("No. Of Decimal Places (6)"=u32 1, "Input"=w897) -> ()
        }
        frame Enabled {
        }
      }
      n643 = call-poly <vilib>:"1D String Array to Delimited String.vi"("delimiter"="\r\n", "string array"=w872) -> ("delimited string"=w869:string)  [unwired: 9 in]
      "No. Of Iterations As Block Of Text (easy to copy into Excel)" <- w869
      n644 = invoke class="Application" method="Clipboard.Write"("Param 0"=w869) -> (error out=w870:errorcluster)  [unwired: 3 in, 3 out]
      n645 = call <vilib>:"Clear Errors.vi"("error in (no error)"=w870) -> ()  [unwired: 5 in, 2 out]
      "No. Of Iterations Executed - Loop 1" <- w893
      "Output - Loop 1" <- w895
      "No. Of Iterations Executed - Loop 2" <- w892
      "Output - Loop 2" <- w894
      "No. Of Iterations Executed - Loop 3" <- w888
      "Output - Loop 3" <- w890
      "No. Of Iterations Executed - Loop 4" <- w887
      "Output - Loop 4" <- w889
      "No. Of Iterations Executed - Loop 5" <- w879
      "Output - Loop 5" <- w885
      "No. Of Iterations Executed - Loop 6" <- w878
      "Output - Loop 6" <- w884
      "No. Of Iterations Executed - Loop 7" <- w877
      "Output - Loop 7" <- w883
      "No. Of Iterations Executed - Loop 8" <- w876
      "Output - Loop 8" <- w882
      "No. Of Iterations Executed - Loop 9" <- w875
      "Output - Loop 9" <- w881
      "No. Of Iterations Executed - Loop 10" <- w874
      "Output - Loop 10" <- w880
      "No. Of Iterations Executed - Loop 11" <- w864
      "Output - Loop 11" <- w868
      "No. Of Iterations Executed - Loop 12" <- w863
      "Output - Loop 12" <- w867
      "No. Of Iterations Executed - Loop 13" <- w862
      "Output - Loop 13" <- w866
      "No. Of Iterations Executed - Loop 14" <- w861
      "Output - Loop 14" <- w865
    }
  }
